vi "Preference_Panel.vi"(0 "Mode":T1) -> ()   [LabVIEW 2011]
uses:
  Anemometry Sub Vis/Controls/Server_Comms.ctl
  Anemometry Sub Vis/Controls/Preference_Mode.ctl
  Anemometry Sub Vis/File/Setup_Filetype.ctl
  Anemometry Sub Vis/Controls/Overhead.ctl
  <vilib>/Instr/_visa.llb/VISA Find Search Mode.ctl
  ADAM Client/Sub VIs/ADAM Controls/Calib_type_ADAM.ctl
  ADAM Client/Sub VIs/ADAM Controls/Module_type_ADAM.ctl
  ADAM Client/Sub VIs/ADAM Controls/Ch_description_ADAM.ctl
  ADAM Client/Sub VIs/ADAM Controls/Function_ADAM.ctl
  ADAM Client/Sub VIs/ADAM Controls/Channel_State.ctl
  ADAM Client/Sub VIs/ADAM Controls/Address.ctl
  Anemometry Sub Vis/Globals/Constants_global.vi
  Anemometry Sub Vis/Globals/Preference_global.vi
  Anemometry Sub Vis/Globals/Trav_pos_global.vi
  Anemometry Sub Vis/Globals/Qnet_Globals.vi
  Anemometry Sub Vis/Acquisition/PWA/PWAtasksGLOBAL.vi
  Anemometry Sub Vis/Globals/Dynamic_call_global.ph.vi
panel:
  in  "Post Processing Machine":bool
  in  "Analogue Device Serial No.":string="1188AB4"
  in  "PWA Device Serial No.":string="1187C98"
  in  "ADAM Setup File":u16(ring) items=["Scani_Valve.xls", "Current_Setup.xls"]
  in  "Default Source Establishment Time (s)":dbl=20.0
  out "This Machine's IP Number":string
  in  "Rig Setup":u16(ring) items=["3_x_2_tunnel", "A_Tunnel", "Adam_Sayer_Desk", "ADAM_Server", "Aero_Tunnel", "Alex_Desktop", "B_Tunnel", "Calibration_Tunnel", "Contact_Conductance", "D_Tunnel", "EnFlo_Tunnel", "Frauke_Desktop", "Fruit_Rig", "iMac_G5_2", "iMacDuo1", "Matteo's_desktop", "Matteo_PC", "Nick_PC-2", "Paul_Desk-Paul_Desk_Machine", "Paul_Hayden-Desk", "Paul_N_Desk_Machine_2", "phtest", "Post_Processing_Machine", "PowerBook_G4_1", "PowerBook_G4_2", "Syn_jet_rig", "Tank", "tdf", "Tom_Desk", "Towing_tank", "--New Rig Setup--"]
  in  "Default Traverse Name":u16(ring) items=["A_Tunnel", "Aero_Laser", "Aero_ThroughWall", "Aero_Tunnel", "Angle_Calibrator", "B_Tunnel", "D_Tunnel", "Dummy_Traverse", "EnFlo_Stack", "EnFlo_Tunnel", "EnFlo_Turntable", "Laser_Meas_Traverse", "mohd_setup", "Paul_Desk_Test", "PIV_Traverse", "--New Traverse Setup--"]
  in  "OK":bool
  in  "% Error From First Calib":dbl=10.0 format="%.1f"
  in  "% Error From Previous Calib":dbl=0.5 format="%.1f"
  in  "Qnet Site Root":path=path "/G4_2_HD/Users/paulhayden/Qnet/qnet"
  out "Templates":path=path "/G4_2_HD/Applications (Mac OS 9)/EnFlo Software/Anemometry/Anemometry Sub Vis/Templates"
  in  "Data Folder":path
  out "EnFlo SW Preferences":path=path "/G4_2_HD/Applications (Mac OS 9)/LabVIEW 5.1/EnFlo SW Preferences"
  in  "Tunnel Speed Control":bool
  in  "SMTP server IP address":string
  in  "Abs Press (mbar)":string="Froude:NPL:Atmos_Press"
  in  "Temperature":string="EnFlo Tun:Inlet Heater:Av Temp"
  in  "Server port number":u32=3363
  in  "Server address":string
  in  "LabVIEW Administrators":string[](array[string])=["", "", "", "", "", "", "", "", "", "", "", "", "", "", "", "", "", "", "", ""]
  in  "Server Comms":T2=enum."Do Not Link To Server"
  # "Server Computer Peferences"
  # "Multi Run Preferences"
  # "Warning Levels for Autocalibration Changes"
  # "Email Peferences"
  # "Deg C"
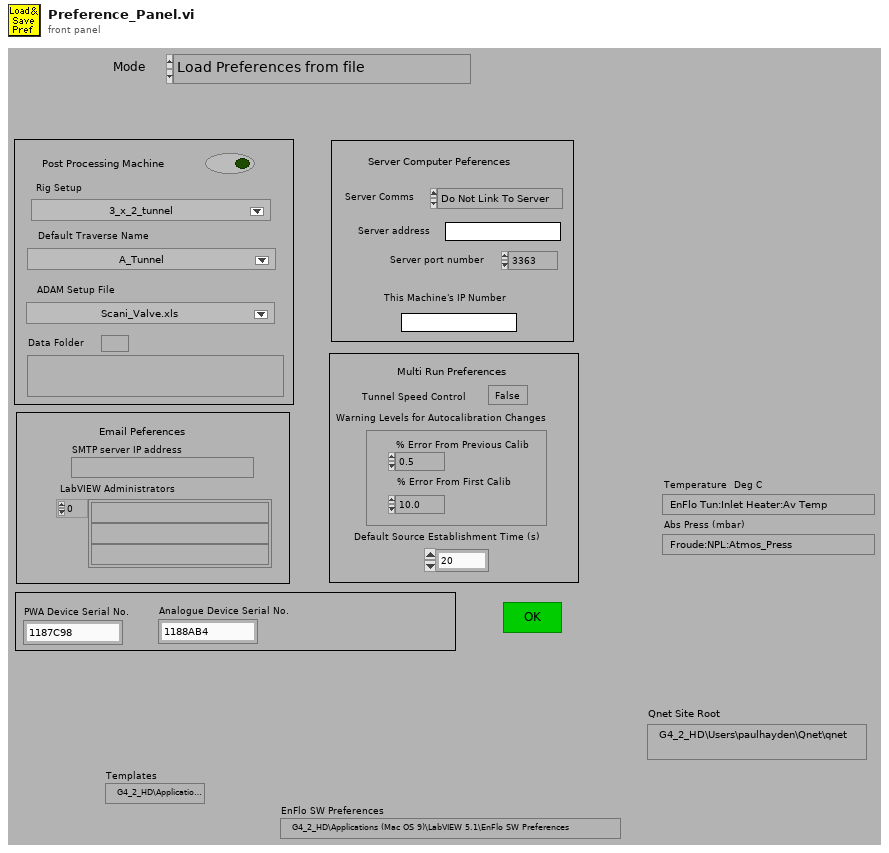
[diagram p1: front panel]
types:
  T1 = typedef "Preference_Mode.ctl" = enum16{"Load Preferences from file", "Save Preferences to file", "Load, Edit then Save"}
  T2 = typedef "Server_Comms.ctl" = enum16{"Server Link Healthy", "Do Not Link To Server"}
  T3 = enum8{"Enabled", "Disabled", "Disabled and Grayed Out"}
  T4 = enum16{"Zero or one", "One", "Zero or more", "One or more"}
  T5 = typedef "Setup_Filetype.ctl" = enum16{"Measurement Setups", "Calibration Setups", "General", "Results File Plotter Setups", "Speed Calib Tweaks"}
  T6 = typedef "Overhead.ctl" = enum16{"Update total times", "Read Current Overhead", "Re Scale totals to 3 hrs", "Initialise totals to 3hr"}
  T7 = typedef "Calib_type_ADAM.ctl" = enum16{"Raw", "Bx + A", "Cx^2 + Bx + A", "Dx^3 + Cx^2 + Bx + A", "In Band", "Hi-Tec Q", "Hi-Tec M_dot", "Text"}
  T8 = typedef "Module_type_ADAM.ctl" = enum16{"4011", "4012", "4013", "4014", "4016", "4017", "4018", "4021", "4050", "4052", "4053", "4060", "4080", "5000", "5017", "5018", "5024", "5051", "5056", "5060", "6060", "Tracker", "WEST", "GILL", "JEM", "VICI", "Vaisala", "DRUCK", "Run VI Named:", "IR2100", "PPT", "Comparator", "VIRTUAL", "Hold Value", "Read A", "Read Ch", "Coded", "Client Info", "Web Client", "X10", "Test"}
  T9 = typedef "Channel_State.ctl" = enum16{"On", "Off", "Always On", "Always Off"}
  T10 = typedef "LVDateTimeRec.ctl" = cluster{"fractional second":dbl, "second":i32, "minute":i32, "hour":i32, "day of month":i32, "month":i32, "year":i32, "day of week":i32, "day of year":i32, "DST":i32}
  T11 = typedef "VISA Find Search Mode.ctl" = u32
  T12 = typedef "Ch_description_ADAM.ctl" = cluster{"Ch Name":string, "Type":T8, "Function":T13, "Ch State":T9, "Calibration type":T7, "A":dbl, "B":dbl, "C":dbl, "D":dbl, "Comments":string, "Address":T14, "String":string, "Duty":u16}
  T13 = typedef "Function_ADAM.ctl" = enum16{"Analogue Input", "Digital Input", "Event counter", "Event rate", "Analogue Output", "Digital Output", "Relay Output"}
  T14 = typedef "Address.ctl" = cluster{"Main":i32, "Ch.":i32, "Sub":i32, "Port Name":string}
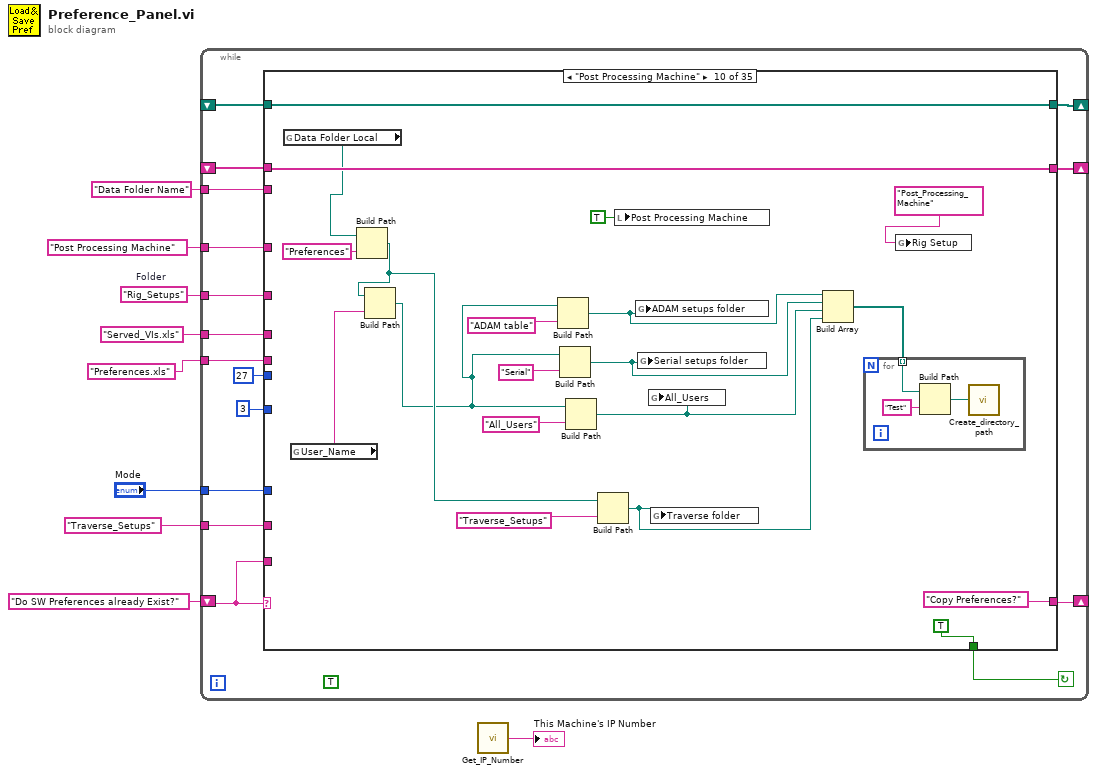
[diagram p0: block diagram]
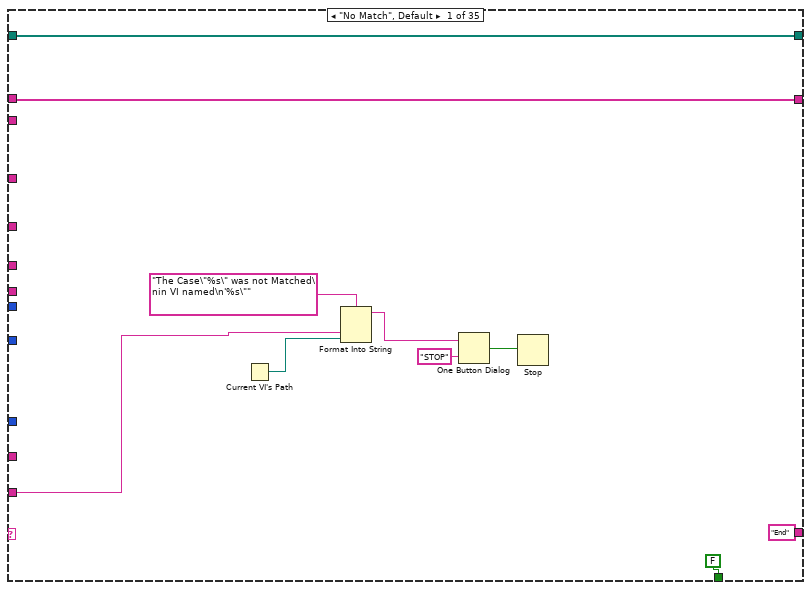
[diagram p2: hidden frame]
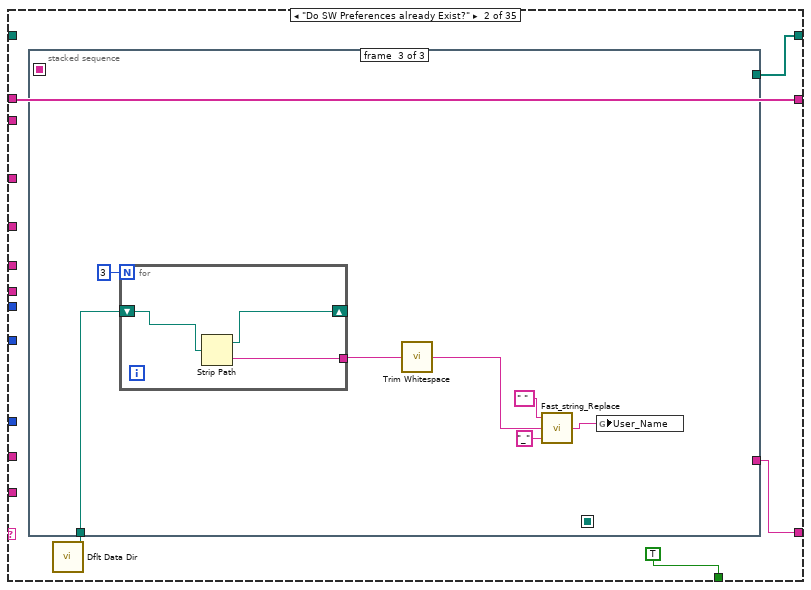
[diagram p3: hidden frame]
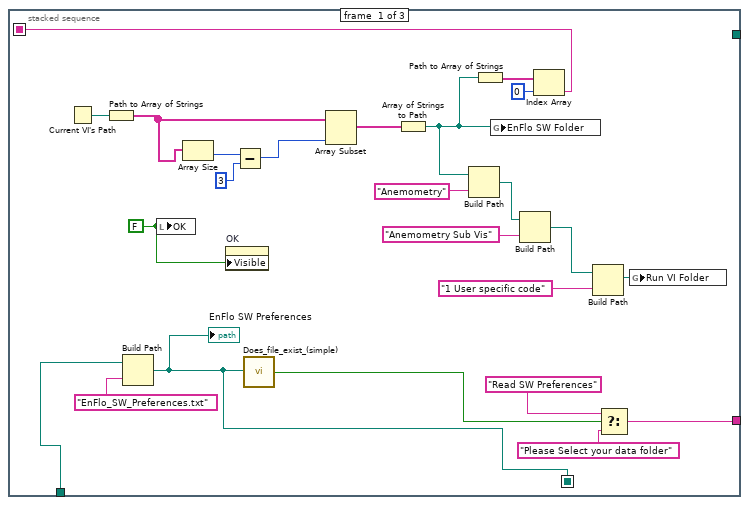
[diagram p4: hidden frame]
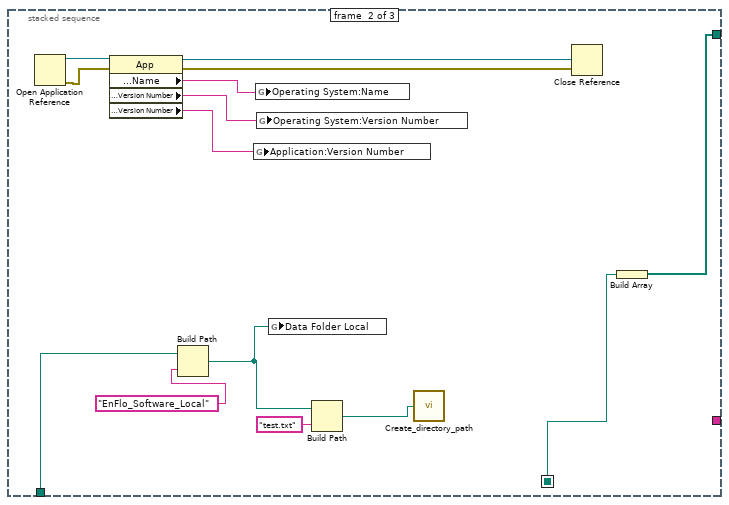
[diagram p5: hidden frame]
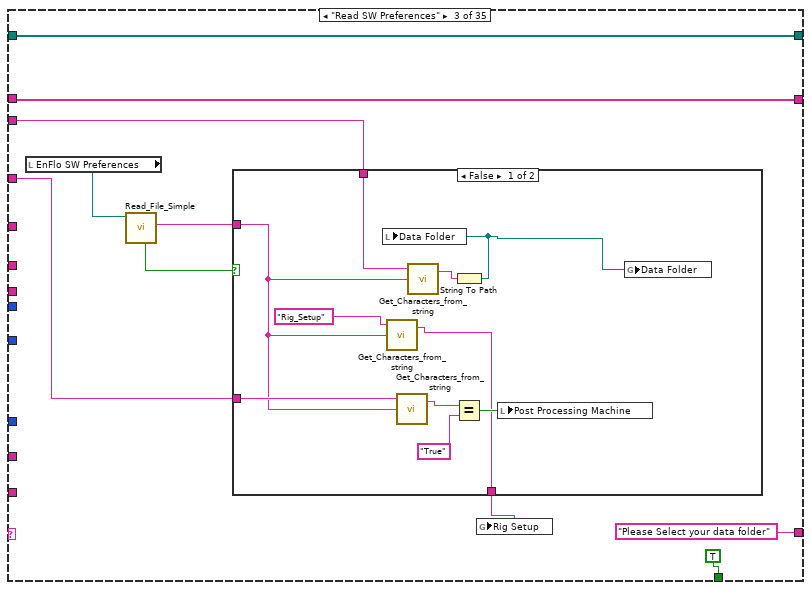
[diagram p6: hidden frame]
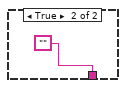
[diagram p7: hidden frame]
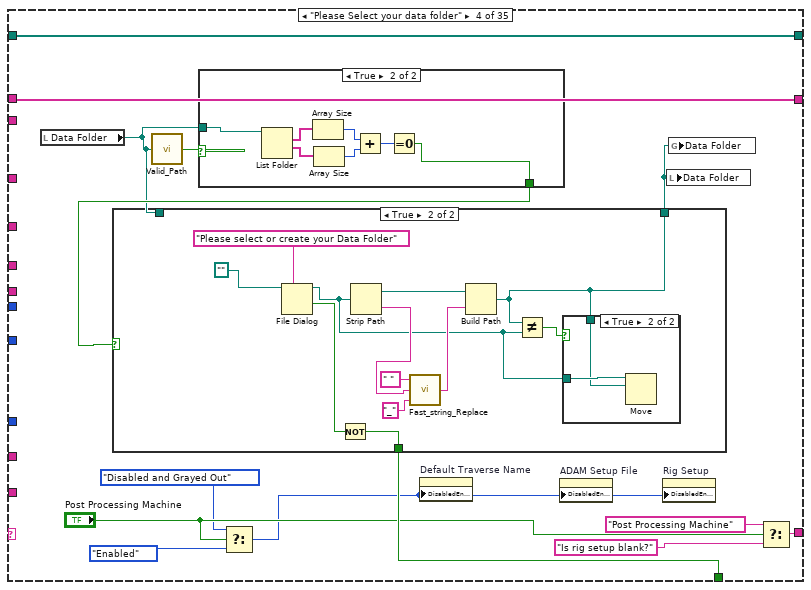
[diagram p8: hidden frame]
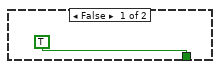
[diagram p9: hidden frame]
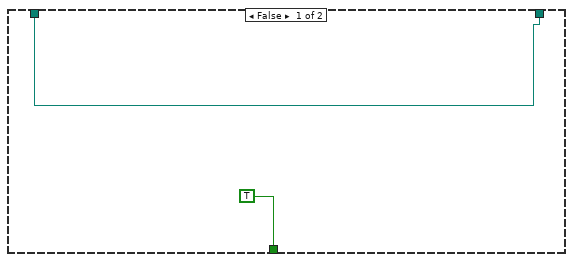
[diagram p10: hidden frame]
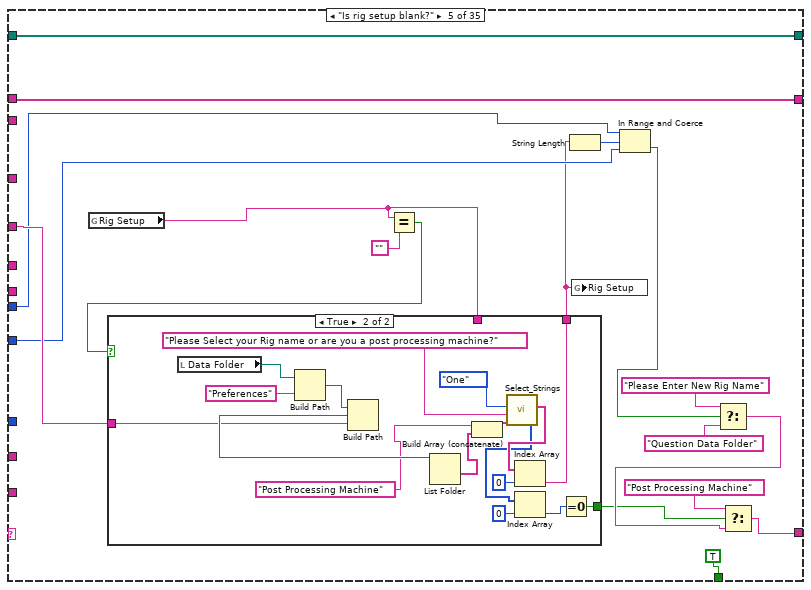
[diagram p12: hidden frame]
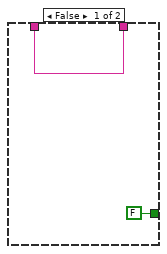
[diagram p13: hidden frame]
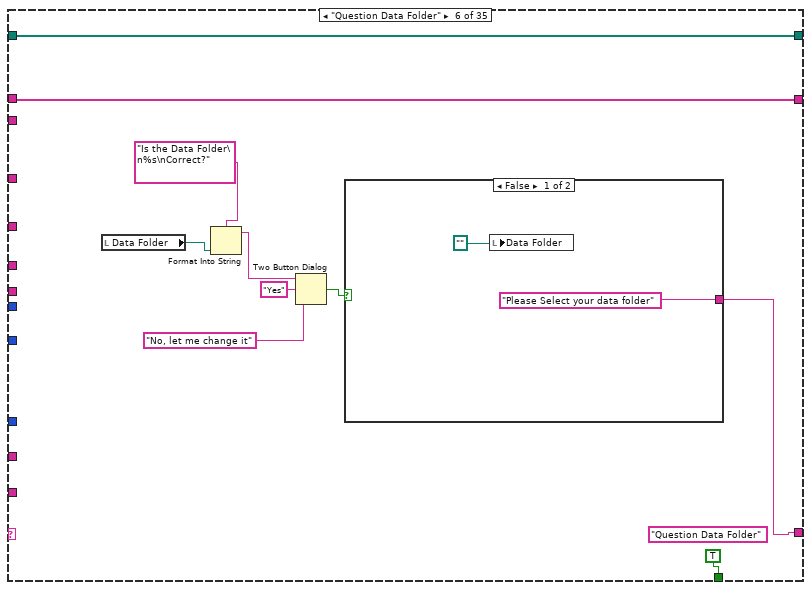
[diagram p14: hidden frame]
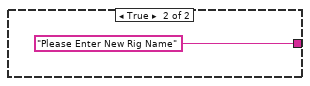
[diagram p15: hidden frame]
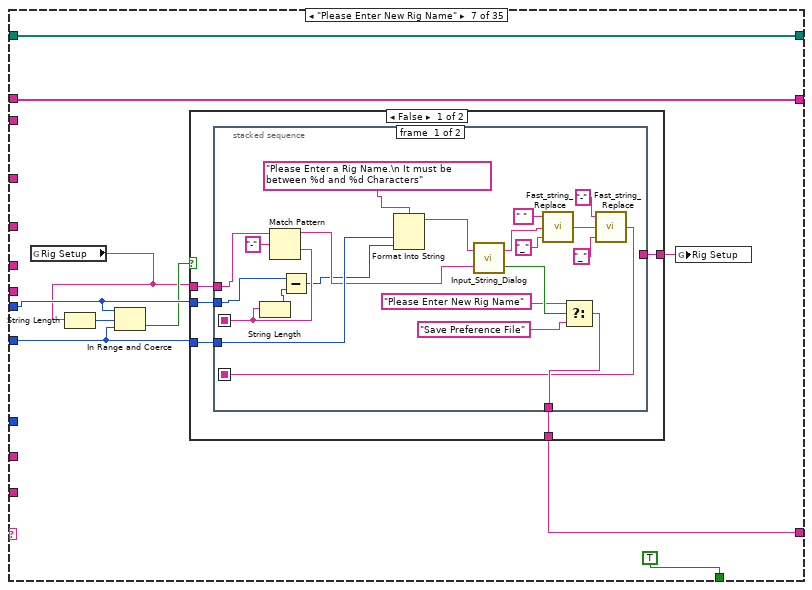
[diagram p16: hidden frame]
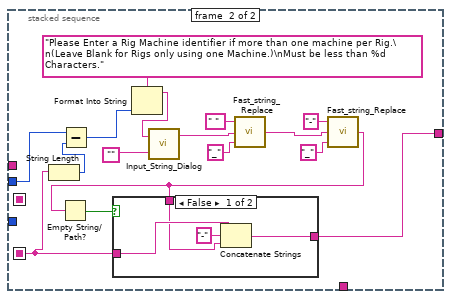
[diagram p17: hidden frame]
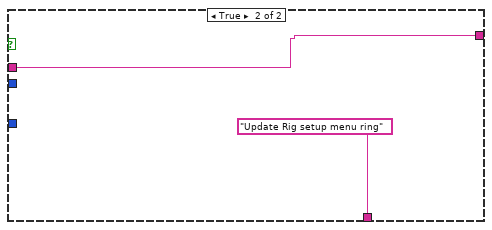
[diagram p19: hidden frame]
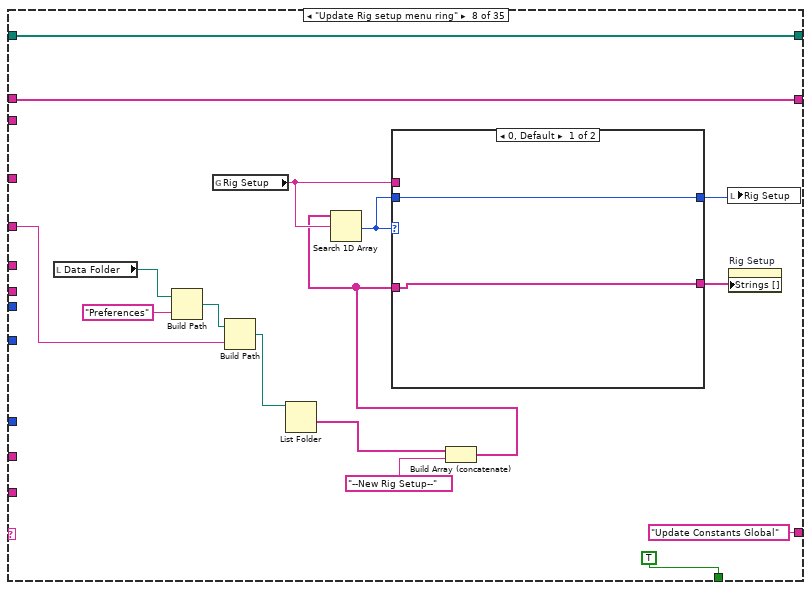
[diagram p20: hidden frame]
diagram:
  w4 = "Rig_Setups"  # Folder
  n1 = while {
    shift-left: _ -> [w22]
    shift-right: [w23] -> _
    shift-left: "Do SW Preferences already Exist?" -> [w10]
    shift-right: [w24] -> _
    tunnel: "Mode" -> [w21]
    tunnel: "Data Folder Name" ("Label for characters") -> [w20]
    tunnel: "Served_VIs.xls" ("Substring") -> [w19]
    tunnel: "Preferences.xls" ("name or relative path") -> [w18]
    tunnel: w4 -> [w15]
    tunnel: "Traverse_Setups" ("name or relative path") -> [w14]
    shift-right: [w13] -> _
    shift-left: _ -> [w12]
    tunnel: "Post Processing Machine" ("Label for characters") -> [w11]
    stop <- w25 continue-if-true
    (unwired) TRUE ("append to file? (new file:F)")
    n2 = case shown="\"Post Processing Machine\"" w10 {
      tunnel: [FALSE TRUE TRUE w117 TRUE TRUE TRUE TRUE TRUE TRUE TRUE TRUE TRUE TRUE TRUE TRUE TRUE TRUE TRUE TRUE TRUE TRUE TRUE TRUE TRUE TRUE TRUE TRUE TRUE TRUE w881 TRUE TRUE TRUE FALSE] -> w25
      tunnel: ["End" w38 "Please Select your data folder" w114 w149 w185 w204 "Update Constants Global" ("f") "Copy Preferences?" "Copy Preferences?" w332 w342 "Install Preference files" "Install Adam table files" "Install Adam setup files" "Choose ADAM Setup file" "Preference files continued" "Variable Names" w517 w537 "Please Enter new  Traverse Setup" w609 "Create Traverse setup" ("f") "Check file permission status" w706 w737 w757 w776 w793 "Save Preference File" "Save SW Preferences" w945 w958 "Initialise Globals" "End"] -> w24
      tunnel: [w27 w39 w97 w123 w164 w193 w206 w271 w297 w320 w330 w347 w405 w420 w445 w464 w486 w496 w522 w544 w597 w611 w645 w662 w707 w742 w762 w785 w798 w812 w887 w953 w959 w1011 w1071] -> w23
      tunnel: w22 -> [w27 w39 w97 w123 w164 w193 w206 w271 w297 w320 w330 w347 w405 w420 w445 w464 w486 w496 _ w544 w597 w611 w645 w662 w707 w742 w762 w785 w798 w812 w887 w953 w959 w1011 w1071]
      tunnel: w10 -> [w30 _ _ _ _ _ _ _ _ _ _ _ _ _ _ _ _ _ _ _ _ _ _ _ _ _ _ _ _ _ _ _ _ _ _]
      tunnel: w21 -> [_ _ _ _ _ _ _ _ _ _ _ _ _ _ _ _ _ _ w516 _ _ _ _ _ w705 _ _ _ _ _ w882 _ _ _ _]
      tunnel: w20 -> [_ _ w94 _ _ _ _ _ _ _ _ _ _ _ _ _ _ _ _ _ _ _ _ _ _ _ _ _ _ _ _ w944 _ _ _]
      tunnel: w19 -> [_ _ _ _ _ _ _ _ _ _ _ _ _ w415 _ _ _ _ _ _ _ _ _ _ _ _ _ _ _ _ _ _ _ w1003 _]
      tunnel: w18 -> [_ _ _ _ _ _ _ _ _ _ w326 w346 _ _ _ _ _ _ _ w534 _ _ _ _ _ _ _ _ _ _ w878 _ _ _ _]
      tunnel: 3 ("lower limit") -> [_ _ _ _ w156 _ w203 _ _ _ _ _ _ _ _ _ _ _ _ _ _ w608 _ _ _ _ _ _ _ _ _ _ _ _ _]
      tunnel: 27 ("upper limit") -> [_ _ _ _ w157 _ w202 _ _ _ _ _ _ _ _ _ _ _ _ _ _ w607 _ _ _ _ _ _ _ _ _ _ _ _ _]
      tunnel: w15 -> [_ _ _ _ w161 _ _ w259 w285 _ _ w345 _ _ _ _ _ _ _ _ _ _ _ _ _ _ _ _ _ _ _ _ _ _ _]
      tunnel: w14 -> [_ _ _ _ _ _ _ _ _ _ _ _ _ _ _ _ _ _ _ _ w595 _ w632 _ _ _ _ _ _ w811 _ _ _ _ _]
      tunnel: [w26 w36 w93 w118 w159 w192 w198 w257 w282 w309 w331 w348 w398 w411 w438 w461 w472 w488 w509 w540 w594 w603 w631 w658 path[] [] w734 w754 w779 w796 w810 w880 w941 w957 w1005 w1068] -> w13
      tunnel: w12 -> [w26 _ w93 w118 w159 w192 w198 w257 w282 w309 w331 w348 w397 w413 w438 w462 w472 w490 w509 w541 w594 w603 w631 w659 w704 w734 w754 w779 w796 w810 w880 w941 w957 w1005 w1068]
      tunnel: w11 -> [_ _ w92 _ _ _ _ _ _ _ _ _ _ _ _ _ _ _ _ _ _ _ _ _ _ _ _ _ _ _ _ w935 _ _ _]
      frame "No Match", Default {
        n3 = Current VI's Path() -> (path=w35:path)
        n4 = Format Into String(format string="The Case\"%s\" was not Matched\nin VI named\n'%s\"" ("Format String"), w30, w35) -> (resulting string=w32:string)  [unwired: 2 in, 1 out]
        n5 = One Button Dialog(message=w32, button name ("OK")="STOP") -> (true=w34:bool)
        n6 = Stop(stop? (T)=w34) -> ()
      }
      frame "Do SW Preferences already Exist?" {
        n7 = call <vilib>:"Dflt Data Dir.vi"() -> ("App:Default Data Directory"=w37:path)
        n8 = stacked-sequence {
          seq-local: [w44 _ _] -> [_ _ _]
          seq-local: [w42 _ _] -> [_ w70 _]
          tunnel: [w48 _ _] -> w38
          tunnel: w37 -> [w43 w68 w84]
          tunnel: [_ w71 _] -> w36
          frame #0 {
            w41 = FALSE ("OK")
            n9 = Current VI's Path() -> (path=w62:path)
            n10 = Path to Array of Strings(0:w62) -> (2:w59:string[])  [unwired: 1 out]
            n11 = Build Path(base path=w43, name or relative path="EnFlo_SW_Preferences.txt") -> (appended path=w42:path)
            "EnFlo SW Preferences" <- w42
            n12 = local write "OK"(w41) -> ()
            n13 = Array Size(array=w59) -> (size(s)=w61:i32)
            n14 = property on="OK" class="Bool (strict)"("Visible"=w41) -> ()  [unwired: 2 in, 2 out]
            n15 = Subtract(x=w61, y=3) -> (x-y=w57:i32)
            n16 = call "Does_file_exist_(simple).vi"("Pathname"=w42) -> ("exists?"=w63:bool)
            n17 = Array Subset(array=w59, length=w57) -> (w58:string[])  [unwired: 1 in]
            n18 = Array of Strings to Path(0:w58) -> (2:w45:path)  [unwired: 1 out]
            n19 = Build Path(base path=w45, name or relative path="Anemometry") -> (appended path=w54:path)
            n20 = Path to Array of Strings(0:w45) -> (2:w46:string[])  [unwired: 1 out]
            n21 = global write "Constants_global.vi" "EnFlo SW Folder"(w45) -> ()
            n22 = Build Path(base path=w54, name or relative path="Anemometry Sub Vis") -> (appended path=w52:path)
            n23 = Index Array(array=w46, index=0) -> (element=w44:string)
            n24 = Build Path(base path=w52, name or relative path="1 User specific code") -> (appended path=w51:path)
            n25 = Select(t="Read SW Preferences", s=w63, f="Please Select your data folder") -> (s? t:f=w48:string)
            n26 = global write "Constants_global.vi" "Run VI Folder"(w51) -> ()
          }
          frame #1 {
            n27 = Open Application Reference() -> (0:w75:errorcluster, 3:w78:refnum<vi>)  [unwired: 1 in, 3 out]
            n28 = property class="App"(reference=w78, error in=w75) -> (reference out=w77:refnum<vi>, error out=w76:errorcluster, "Operating System:Name"=w72:string, "Operating System:Version Number"=w74:string, "Application:Version Number"=w73:string)
            n29 = Build Path(base path=w68, name or relative path="EnFlo_Software_Local" ("element")) -> (appended path=w67:path)
            n30 = global write "Preference_global.vi" "Application:Version Number"(w73) -> ()
            n31 = global write "Preference_global.vi" "Operating System:Name"(w72) -> ()
            n32 = global write "Preference_global.vi" "Operating System:Version Number"(w74) -> ()
            n33 = global write "Constants_global.vi" "Data Folder Local"(w67) -> ()
            n34 = Build Path(base path=w67, name or relative path="test.txt") -> (appended path=w65:path)
            n35 = call "Create_directory_path.vi"("Path name"=w65) -> ()  [unwired: 1 out]
            n36 = Close Reference(reference=w77, error in (no error)=w76) -> ()  [unwired: 1 out]
            n37 = Build Array(w70) -> (w71:path[])
          }
          frame #2 {
            n38 = for {
              N: 3 -> [_]
              shift-right: [w88] -> _
              shift-left: w84 -> [w87]
              tunnel: [w86] -> w80
              n39 = Strip Path(path=w87) -> (stripped path=w88:path, name=w86:string)
            }
            n40 = call <vilib>:"Trim Whitespace.vi"("string"=w80) -> ("trimmed string"=w79:string)  [unwired: 1 in]
            n41 = call "Fast_string_Replace.vi"("Replace match with:"="_", "Input String"=w79, "regular expression"=" ") -> ("Output String"=w81:string)  [unwired: 1 in, 1 out]
            n42 = global write "Preference_global.vi" "User_Name"(w81) -> ()
          }
        }
      }
      frame "Read SW Preferences" {
        n43 = local read "EnFlo SW Preferences"() -> (w96:path)
        n44 = call "Read_File_Simple.vi"("Filename"=w96) -> ("Error?"=w90:bool, "string"=w91:string)  [unwired: 2 in, 6 out]
        n45 = case shown="False" w90 {
          tunnel: w94 -> [w107 _]
          tunnel: w92 -> [w104 _]
          tunnel: w91 -> [w103 _]
          tunnel: [w99 ""] -> w89
          frame False {
            n46 = call "Get_Characters_from_string.vi"("Input string"=w103, "Variable name"="Rig_Setup" ("Label for characters")) -> ("Value"=w99:string)  [unwired: 1 in, 1 out]
            n47 = call "Get_Characters_from_string.vi"("Input string"=w103, "Variable name"=w104) -> ("Value"=w102:string)  [unwired: 1 in, 1 out]
            n48 = call "Get_Characters_from_string.vi"("Input string"=w103, "Variable name"=w107) -> ("Value"=w108:string)  [unwired: 1 in, 1 out]
            n49 = String To Path(string=w108) -> (path=w106:path)
            n50 = local write "Data Folder"(w106) -> ()
            n51 = Equal?(x=w102, y="True") -> (x = y?=w100:bool)
            n52 = local write "Post Processing Machine"(w100) -> ()
            n53 = global write "Constants_global.vi" "Data Folder"(w106) -> ()
          }
          frame True {
          }
        }
        n54 = global write "Preference_global.vi" "Rig Setup"(w89) -> ()
      }
      frame "Please Select your data folder" {
        n55 = local read "Data Folder"() -> (w119:path)
        n56 = call "Valid_Path.vi"("Filename"=w119) -> ("Valid Path?"=w121:bool)
        n57 = case shown="True" w121 {
          tunnel: [TRUE ("status") w125] -> w120
          tunnel: w119 -> [_ w131]
          frame False {
          }
          frame True {
            n58 = List Folder(path=w131) -> (filenames=w129:string[], folder names=w130:string[])  [unwired: 1 in, 4 out]
            n59 = Array Size(array=w129) -> (size(s)=w127:i32)
            n60 = Array Size(array=w130) -> (size(s)=w128:i32)
            n61 = Add(x=w127, y=w128) -> (x+y=w126:i32)
            n62 = Equal To 0?(x=w126) -> (x = 0?=w125:bool)
          }
        }
        n63 = case shown="True" w120 {
          tunnel: [w133 w136] -> w122
          tunnel: w119 -> [w133 _]
          tunnel: [TRUE w134] -> w117
          frame False {
          }
          frame True {
            n64 = File Dialog(7:"Please select or create your Data Folder" ("prompt"), 11:path "") -> (1:w135:bool, 3:w137:path)  [unwired: 1 in, 6 out]
            n65 = Not(x=w135) -> (.not. x?=w134:bool)
            n66 = Strip Path(path=w137) -> (stripped path=w141:path, name=w140:string)
            n67 = call "Fast_string_Replace.vi"("Replace match with:"="_", "Input String"=w140, "regular expression"=" ") -> ("Output String"=w139:string)  [unwired: 2 out]
            n68 = Build Path(base path=w141, name or relative path=w139) -> (appended path=w136:path)
            n69 = Not Equal?(x=w136, y=w137) -> (x != y?=w138:bool)
            n70 = case shown="True" w138 {
              tunnel: w137 -> [_ w147]
              tunnel: w136 -> [_ w146]
              frame False {
              }
              frame True {
                n71 = Move(source path=w147, 10:w146) -> ()  [unwired: 1 in, 5 out]
              }
            }
          }
        }
        n72 = Select(t=T3."Disabled and Grayed Out" ("Disabled"), s="Post Processing Machine", f=T3."Enabled" ("Disabled")) -> (s? t:f=w110:T3)
        n73 = property on="Default Traverse Name" class="Ring (strict)"("DisabledEnum"=w110) -> ()  [unwired: 2 in, 2 out]
        n74 = property on="ADAM Setup File" class="Ring (strict)"("DisabledEnum"=w110) -> ()  [unwired: 2 in, 2 out]
        n75 = property on="Rig Setup" class="Ring (strict)"("DisabledEnum"=w110) -> ()  [unwired: 2 in, 2 out]
        n76 = local write "Data Folder"(w122) -> ()
        n77 = global write "Constants_global.vi" "Data Folder"(w122) -> ()
        n78 = Select(t="Post Processing Machine", s="Post Processing Machine", f="Is rig setup blank?") -> (s? t:f=w114:string)
      }
      frame "Is rig setup blank?" {
        n79 = global read "Preference_global.vi" "Rig Setup"() -> (w160:string)
        n80 = Equal?(x=w160, y="") -> (x = y?=w162:bool)
        n81 = case shown="True" w162 {
          tunnel: w161 -> [_ w180]
          tunnel: [w167 w178] -> w155
          tunnel: w160 -> [w167 _]
          tunnel: [FALSE w168] -> w148
          frame False {
          }
          frame True {
            n82 = local read "Data Folder"() -> (w183:path)
            n83 = Build Path(base path=w183, name or relative path="Preferences") -> (appended path=w182:path)
            n84 = Build Path(base path=w182, name or relative path=w180) -> (appended path=w181:path)
            n85 = List Folder(path=w181) -> (folder names=w175:string[])  [unwired: 1 in, 5 out]
            n86 = Build Array (concatenate)("Post Processing Machine", w175) -> (w173:string[])
            n87 = call "Select_Strings.vi"("Available Ch names"=w173, "Message"="Please Select your Rig name or are you a post processing machine?", "Selector mode"=T4."One") -> ("Ch Indicies Choosen"=w170:i32[], "Selected Channel Names"=w172:string[])  [unwired: 3 in, 1 out]
            n88 = Index Array(array=w172, index=0) -> (element=w178:string)
            n89 = Index Array(array=w170, index=0) -> (element=w169:i32)
            n90 = Equal To 0?(x=w169) -> (x = 0?=w168:bool)
          }
        }
        n91 = String Length(string=w155) -> (length=w158:i32)
        n92 = global write "Preference_global.vi" "Rig Setup"(w155) -> ()
        n93 = In Range and Coerce(upper limit=w157, x=w158, lower limit=w156) -> (In Range?=w154:bool)  [unwired: 1 out]
        n94 = Select(t="Please Enter New Rig Name", s=w154, f="Question Data Folder") -> (s? t:f=w150:string)
        n95 = Select(t="Post Processing Machine", s=w148, f=w150) -> (s? t:f=w149:string)
      }
      frame "Question Data Folder" {
        (unwired) "Question Data Folder"
        n96 = local read "Data Folder"() -> (w191:path)
        n97 = Format Into String(format string="Is the Data Folder\n%s\nCorrect?" ("message"), w191) -> (resulting string=w189:string)  [unwired: 2 in, 1 out]
        n98 = Two Button Dialog(message=w189, 1:"No, let me change it" ("F button name (\"Cancel\")"), 2:"Yes" ("T button name (\"OK\")")) -> (T button?=w186:bool)
        n99 = case shown="False" w186 {
          tunnel: ["Please Select your data folder" "Please Enter New Rig Name"] -> w185
          frame False {
            n100 = local write "Data Folder"(path "") -> ()
          }
          frame True {
          }
        }
      }
      frame "Please Enter New Rig Name" {
        n101 = global read "Preference_global.vi" "Rig Setup"() -> (w200:string)
        n102 = String Length(string=w200) -> (length=w205:i32)
        n103 = In Range and Coerce(upper limit=w202, x=w205, lower limit=w203) -> (In Range?=w201:bool)  [unwired: 1 out]
        n104 = case shown="False" w201 {
          tunnel: w200 -> [w212 w255]
          tunnel: [w208 "Update Rig setup menu ring"] -> w204
          tunnel: [w209 w255] -> w199
          tunnel: w203 -> [w211 _]
          tunnel: w202 -> [w210 _]
          frame False {
            n105 = stacked-sequence {
              seq-local: [w213 _] -> [_ w238]
              seq-local: [w220 _] -> [_ _]
              tunnel: w212 -> [w222 _]
              tunnel: w211 -> [w233 _]
              tunnel: w210 -> [w219 w236]
              tunnel: [_ w241] -> w209
              tunnel: [w225 _] -> w208
              frame #0 {
                n106 = Match Pattern(string=w222, regular expression="-") -> (before substring=w221:string, after substring=w220:string)  [unwired: 3 out]
                n107 = String Length(string=w220) -> (length=w218:i32)
                n108 = Subtract(x=w219, y=w218) -> (x-y=w217:i32)
                n109 = Format Into String(format string="Please Enter a Rig Name.\n It must be between %d and %d Characters" ("Message to user"), w233, w217) -> (resulting string=w232:string)  [unwired: 2 in, 1 out]
                n110 = call "Input_String_Dialog.vi"("Value"=w221, "Message to user"=w232) -> ("Ok Out"=w228:bool, "Output string"=w229:string)
                n111 = call "Fast_string_Replace.vi"("Replace match with:"="_", "Input String"=w229, "regular expression"=" ") -> ("Output String"=w214:string)  [unwired: 2 out]
                n112 = Select(t="Please Enter New Rig Name", s=w228, f="Save Preference File") -> (s? t:f=w225:string)
                n113 = call "Fast_string_Replace.vi"("Replace match with:"="_", "Input String"=w214, "regular expression"="-") -> ("Output String"=w213:string)  [unwired: 2 out]
              }
              frame #1 {
                n114 = String Length(string=w238) -> (length=w237:i32)
                n115 = Subtract(x=w236, y=w237) -> (x-y=w235:i32)
                n116 = Format Into String(format string="Please Enter a Rig Machine identifier if more than one machine per Rig.\n(Leave Blank for Rigs only using one Machine.)\nMust be less than %d Characters." ("Message to user"), w235) -> (resulting string=w234:string)  [unwired: 2 in, 1 out]
                n117 = call "Input_String_Dialog.vi"("Value"="", "Message to user"=w234) -> ("Output string"=w247:string)  [unwired: 1 out]
                n118 = call "Fast_string_Replace.vi"("Replace match with:"="_", "Input String"=w247, "regular expression"=" ") -> ("Output String"=w243:string)  [unwired: 2 out]
                n119 = call "Fast_string_Replace.vi"("Replace match with:"="_", "Input String"=w243, "regular expression"="-") -> ("Output String"=w240:string)  [unwired: 2 out]
                n120 = Empty String/Path?(string/path=w240) -> (empty?=w242:bool)
                n121 = case shown="False" w242 {
                  tunnel: [w250 w254] -> w241
                  tunnel: w238 -> [w253 w254]
                  tunnel: w240 -> [w251 _]
                  frame False {
                    n122 = Concatenate Strings(w253, "-" ("string"), w251) -> (w250:string)
                  }
                  frame True {
                  }
                }
              }
            }
          }
          frame True {
          }
        }
        n123 = global write "Preference_global.vi" "Rig Setup"(w199) -> ()
      }
      frame "Update Rig setup menu ring" {
        n124 = local read "Data Folder"() -> (w262:path)
        n125 = Build Path(base path=w262, name or relative path="Preferences") -> (appended path=w261:path)
        n126 = global read "Preference_global.vi" "Rig Setup"() -> (w268:string)
        n127 = Build Path(base path=w261, name or relative path=w259) -> (appended path=w260:path)
        n128 = List Folder(path=w260) -> (folder names=w258:string[])  [unwired: 1 in, 5 out]
        n129 = Build Array (concatenate)(w258, "--New Rig Setup--") -> (w264:string[])
        n130 = Search 1D Array(1D array=w264, element=w268) -> (index of element=w267:i32)  [unwired: 1 out]
        n131 = case shown="0, Default" w267 {
          tunnel: [w274 0] -> w270
          tunnel: w264 -> [w273 w277]
          tunnel: w268 -> [_ w276]
          tunnel: w267 -> [w274 _]
          tunnel: [w273 w275] -> w266
          frame 0, Default {
          }
          frame -1 {
            n132 = Build Array (concatenate)(w276, w277) -> (w275:string[])
          }
        }
        n133 = local write "Rig Setup"(w270) -> ()
        n134 = property on="Rig Setup" class="Ring (strict)"("Strings []"=w266) -> ()  [unwired: 2 in, 2 out]
      }
      frame "Update Constants Global" {
        n135 = global read "Constants_global.vi" "Data Folder"() -> (w283:path)
        n136 = global read "Preference_global.vi" "Rig Setup"() -> (w284:string)
        n137 = Build Path(base path=w283, name or relative path="Preferences") -> (appended path=w286:path)
        n138 = Build Path(base path=w286, name or relative path=w285) -> (appended path=w287:path)
        n139 = Build Path(base path=w287, name or relative path=w284) -> (appended path=w279:path)
        n140 = Build Path(base path=w279, name or relative path="ADAM table") -> (appended path=w292:path)
        n141 = Build Path(base path=w279, name or relative path="Serial") -> (appended path=w291:path)
        n142 = Build Path(base path=w279, name or relative path="All_Users") -> (appended path=w280:path)
        n143 = Build Path(base path=w286, name or relative path="Traverse_Setups") -> (appended path=w290:path)
        n144 = global write "Constants_global.vi" "ADAM setups folder"(w292) -> ()
        n145 = global write "Constants_global.vi" "Serial setups folder"(w291) -> ()
        n146 = global write "Constants_global.vi" "All_Users"(w280) -> ()
        n147 = global write "Constants_global.vi" "Traverse folder"(w290) -> ()
        n148 = Build Array(w292, w291, w280, w290) -> (w289:path[])
        n149 = for {
          tunnel: w289 -> [w301] mode=indexing
          n150 = Build Path(base path=w301, name or relative path="Test") -> (appended path=w299:path)
          n151 = call "Create_directory_path.vi"("Path name"=w299) -> ()  [unwired: 1 out]
        }
      }
      frame "Post Processing Machine" {
        n152 = global read "Constants_global.vi" "Data Folder Local"() -> (w308:path)
        n153 = global read "Preference_global.vi" "User_Name"() -> (w303:string)
        n154 = Build Path(base path=w308, name or relative path="Preferences") -> (appended path=w310:path)
        n155 = Build Path(base path=w310, name or relative path=w303) -> (appended path=w304:path)
        n156 = Build Path(base path=w304, name or relative path="ADAM table") -> (appended path=w315:path)
        n157 = Build Path(base path=w304, name or relative path="Serial") -> (appended path=w314:path)
        n158 = Build Path(base path=w304, name or relative path="All_Users") -> (appended path=w305:path)
        n159 = Build Path(base path=w310, name or relative path="Traverse_Setups") -> (appended path=w313:path)
        n160 = local write "Post Processing Machine"(TRUE ("Post Processing Machine")) -> ()
        n161 = global write "Constants_global.vi" "ADAM setups folder"(w315) -> ()
        n162 = global write "Constants_global.vi" "Serial setups folder"(w314) -> ()
        n163 = global write "Constants_global.vi" "All_Users"(w305) -> ()
        n164 = global write "Constants_global.vi" "Traverse folder"(w313) -> ()
        n165 = Build Array(w315, w314, w305, w313) -> (w312:path[])
        n166 = for {
          tunnel: w312 -> [w324] mode=indexing
          n167 = Build Path(base path=w324, name or relative path="Test") -> (appended path=w322:path)
          n168 = call "Create_directory_path.vi"("Path name"=w322) -> ()  [unwired: 1 out]
        }
        n169 = global write "Preference_global.vi" "Rig Setup"("Post_Processing_Machine" ("Rig Setup")) -> ()
      }
      frame "Copy Preferences?" {
        n170 = call "Setup_Filepath.vi"("Setup File Type"=Setup_Filetype."General", "Filename in"=w326) -> ("Filename Out"=w325:path)  [unwired: 1 out]
        n171 = call <vilib>:"Check if File or Folder Exists.vi"("path"=w325) -> ("file or folder exists?"=w329:bool)  [unwired: 1 in, 9 out]
        n172 = case shown="False" w329 {
          tunnel: [w336 TRUE ("Error?")] -> w328
          frame False {
            n173 = global read "Constants_global.vi" "All_Users"() -> (w338:path)
            n174 = Build Path(base path=w338, name or relative path="Current_Username") -> (appended path=w339:path)
            n175 = call "Read_File_Simple.vi"("Filename"=w339) -> ("Error?"=w336:bool)  [unwired: 4 in, 5 out]
          }
          frame True {
          }
        }
        n176 = Select(t="Install Generic Meas Setup file", s=w328, f="Copy from last user") -> (s? t:f=w332:string)
      }
      frame "Copy from last user" {
        n177 = stacked-sequence {
          seq-local: [w359 _ _ _] -> [_ w369 w378 w390]
          seq-local: [_ w364 _ _] -> [_ _ _ w384]
          seq-local: [_ _ w373 _] -> [_ _ _ w383]
          tunnel: w346 -> [_ w367 _ _]
          tunnel: w345 -> [_ _ _ _]
          tunnel: [_ _ _ w382] -> w344
          frame #0 {
            n178 = global read "Constants_global.vi" "All_Users"() -> (w363:path)
            n179 = Seconds To Date/Time() -> (date time rec=w354:T10)  [unwired: 2 out]
            n180 = Unbundle By Name(w354) -> ("year"=w355:i32)
            n181 = global read "Preference_global.vi" "Rig Setup"() -> (w352:string)
            n182 = Build Path(base path=w363, name or relative path="Current_Username") -> (appended path=w361:path)
            n183 = Number To Decimal String(number=w355) -> (decimal integer string=w353:string)  [unwired: 1 out]
            n184 = global read "Constants_global.vi" "Data Folder"() -> (w358:path)
            n185 = call "Read_File_Simple.vi"("Filename"=w361) -> ("string"=w351:string)  [unwired: 4 in, 5 out]
            n186 = Build Path(base path=w358, name or relative path=w353) -> (appended path=w357:path)
            n187 = Build Path(base path=w357, name or relative path=w352) -> (appended path=w356:path)
            n188 = Build Path(base path=w356, name or relative path=w351) -> (appended path=w360:path)
            n189 = Build Path(base path=w360, name or relative path="Preferences") -> (appended path=w359:path)
          }
          frame #1 {
            n190 = call "Setup_Filepath.vi"("Setup File Type"=Setup_Filetype."General", "Filename in"=w367) -> ("Filename Out"=w366:path)  [unwired: 1 out]
            n191 = Build Path(base path=w369, name or relative path="General") -> (appended path=w371:path)
            n192 = Build Path(base path=w371, name or relative path=w367) -> (appended path=w370:path)
            n193 = Copy(10:w366, 11:w370) -> (0:w365:errorcluster)  [unwired: 3 in, 2 out]
            n194 = Unbundle By Name(w365) -> ("status"=w364:bool)
          }
          frame #2 {
            w376 = "Current_Setup.xls"
            n195 = Build Path(base path=w378, name or relative path="Meas Setups") -> (appended path=w380:path)
            n196 = Build Path(base path=w380, name or relative path=w376) -> (appended path=w379:path)
            n197 = call "Setup_Filepath.vi"("Setup File Type"=Setup_Filetype."Measurement Setups", "Filename in"=w376) -> ("Filename Out"=w375:path)  [unwired: 1 out]
            n198 = Copy(10:w375, 11:w379) -> (0:w374:errorcluster)  [unwired: 3 in, 2 out]
            n199 = Unbundle By Name(w374) -> ("status"=w373:bool)
          }
          frame #3 {
            w388 = "Current_Setup.xls"
            n200 = Build Path(base path=w390, name or relative path="Calib Setups") -> (appended path=w392:path)
            n201 = Build Path(base path=w392, name or relative path=w388) -> (appended path=w391:path)
            n202 = call "Setup_Filepath.vi"("Setup File Type"=Setup_Filetype."Calibration Setups", "Filename in"=w388) -> ("Filename Out"=w387:path)  [unwired: 1 out]
            n203 = Copy(10:w387, 11:w391) -> (0:w386:errorcluster)  [unwired: 3 in, 2 out]
            n204 = Unbundle By Name(w386) -> ("status"=w385:bool)
            n205 = Compound Arithmetic op=OR(w385, w384, w383) -> (w382:bool)
          }
        }
        n206 = Select(t="Install Generic Meas Setup file", s=w344, f="Read SW Preferences") -> (s? t:f=w342:string)
      }
      frame "Install Generic Meas Setup file" {
        n207 = global read "Constants_global.vi" "Run VI Folder"() -> (w404:path)
        n208 = Strip Path(path=w404) -> (stripped path=w402:path)  [unwired: 1 out]
        n209 = call "Setup_Filepath.vi"("Setup File Type"=Setup_Filetype."Measurement Setups", "Filename in"="Current_Setup.xls" ("name or relative path")) -> ("Filename Out"=w394:path)  [unwired: 1 out]
        n210 = Build Path(base path=w402, name or relative path="Templates") -> (appended path=w400:path)
        "Templates" <- w400
        n211 = call "Does_file_exist_(simple).vi"("Pathname"=w394) -> ("exists?"=w401:bool)
        n212 = case shown="False" w401 {
          tunnel: w394 -> [w410 _]
          tunnel: w400 -> [w408 _]
          frame False {
            n213 = Build Path(base path=w408, name or relative path="Measurement Setup.xls") -> (appended path=w407:path)
            n214 = Copy(10:w410, 11:w407) -> ()  [unwired: 1 in, 5 out]
          }
          frame True {
          }
        }
        n215 = Build Array (concatenate)(w397, w394) -> (w398:path[])
      }
      frame "Install Preference files" {
        n216 = Build Array("Preferences.xls" ("Substring"), w415, "Month_Names.xls" ("name or relative path"), "LDA_Configuration.xls") -> (w419:string[])
        n217 = for {
          tunnel: w419 -> [w423] mode=indexing
          tunnel: [w422] -> w412 mode=indexing
          n218 = call "Setup_Filepath.vi"("Setup File Type"=Setup_Filetype."General", "Filename in"=w423) -> ("Filename Out"=w422:path)  [unwired: 1 out]
          n219 = call "Does_file_exist_(simple).vi"("Pathname"=w422) -> ("exists?"=w425:bool)
          n220 = case shown="False" w425 {
            tunnel: w422 -> [w429 _]
            tunnel: w423 -> [w426 _]
            frame False {
              n221 = local read "Templates"() -> (w427:path)
              n222 = Build Path(base path=w427, name or relative path=w426) -> (appended path=w428:path)
              n223 = Copy(10:w429, 11:w428) -> ()  [unwired: 1 in, 5 out]
            }
            frame True {
            }
          }
        }
        n224 = Build Array (concatenate)(w413, w412) -> (w411:path[])
      }
      frame "Install Adam table files" {
        w434 = "Current_Setup.xls"
        n225 = global read "Constants_global.vi" "ADAM setups folder"() -> (w436:path)
        n226 = Build Path(base path=w436, name or relative path=w434) -> (appended path=w437:path)
        n227 = Build Path(base path=w436, name or relative path="Setup_Files") -> (appended path=w432:path)
        n228 = Build Array("Hi_Tec_Calibs.xls" ("name or relative path"), "A_Tunnel DB setup.xls" ("Substring"), "EnFlo_Tunnel DB setup.xls", "Aero_Tunnel DB setup.xls" ("name or relative path"), "D_Tunnel DB setup.xls") -> (w444:string[])
        n229 = Build Path(base path=w432, name or relative path=w434) -> (appended path=w431:path)
        n230 = for {
          tunnel: w444 -> [w448] mode=indexing
          tunnel: w436 -> [w449]
          n231 = Build Path(base path=w449, name or relative path=w448) -> (appended path=w447:path)
          n232 = call "Does_file_exist_(simple).vi"("Pathname"=w447) -> ("exists?"=w450:bool)
          n233 = case shown="False" w450 {
            tunnel: w447 -> [w454 _]
            tunnel: w448 -> [w451 _]
            frame False {
              n234 = local read "Templates"() -> (w452:path)
              n235 = Build Path(base path=w452, name or relative path=w451) -> (appended path=w453:path)
              n236 = Copy(10:w454, 11:w453) -> ()  [unwired: 1 in, 5 out]
            }
            frame True {
            }
          }
        }
        n237 = call "Create_directory_path.vi"("Path name"=w431) -> ("Path name Out"=w430:path)
        n238 = Move(source path=w437, 10:w430) -> ()  [unwired: 1 in, 5 out]
      }
      frame "Install Adam setup files" {
        w458 = "Current_Setup.xls"
        n239 = global read "Constants_global.vi" "ADAM setups folder"() -> (w460:path)
        n240 = Build Path(base path=w460, name or relative path="Setup_Files") -> (appended path=w457:path)
        n241 = Build Path(base path=w457, name or relative path=w458) -> (appended path=w455:path)
        n242 = call "Does_file_exist_(simple).vi"("Pathname"=w455) -> ("exists?"=w456:bool)
        n243 = case shown="False" w456 {
          tunnel: w455 -> [w471 _]
          tunnel: w458 -> [w469 _]
          frame False {
            n244 = local read "Templates"() -> (w470:path)
            n245 = Build Path(base path=w470, name or relative path="ADAM_Setup_files") -> (appended path=w468:path)
            n246 = Build Path(base path=w468, name or relative path=w469) -> (appended path=w467:path)
            n247 = Copy(10:w471, 11:w467) -> ()  [unwired: 1 in, 5 out]
          }
          frame True {
          }
        }
        n248 = Build Array (concatenate)(w462, w455) -> (w461:path[])
      }
      frame "Choose ADAM Setup file" {
        w480 = "Selected_Filename.txt" ("Substring")
        n249 = global read "Constants_global.vi" "ADAM setups folder"() -> (w484:path)
        n250 = Build Path(base path=w484, name or relative path="Setup_Files") -> (appended path=w481:path)
        n251 = Build Path(base path=w481, name or relative path=w480) -> (appended path=w479:path)
        n252 = call "Read_File_Simple.vi"("Filename"=w479) -> ("string"=w477:string)  [unwired: 2 in, 7 out]
        n253 = Build Array(w480) -> (w482:string[])
        n254 = call "List_files_in_order_of_age.vi"("Files to Hide"=w482, "Folder"=w481) -> ("file names"=w478:string[])
        n255 = Search 1D Array(1D array=w478, element=w477) -> (index of element=w474:i32)  [unwired: 1 out]
        n256 = property on="ADAM Setup File" class="Ring (strict)"("Strings []"=w478) -> ()  [unwired: 2 in, 2 out]
        n257 = Less Than 0?(x=w474) -> (x < 0?=w475:bool)
        n258 = Select(t=0, s=w475, f=w474) -> (s? t:f=w473:i32)
        n259 = local write "ADAM Setup File"(w473) -> ()
      }
      frame "Preference files continued" {
        n260 = Build Array("Hot_Wire_Bridges.txt", "Hot_Wire_Probes.txt", "Pressure_Transducers.txt") -> (w491:string[])
        n261 = for {
          tunnel: w491 -> [w499] mode=indexing
          tunnel: [w498] -> w489 mode=indexing
          n262 = call "Setup_Filepath.vi"("Setup File Type"=Setup_Filetype."Calibration Setups", "Filename in"=w499) -> ("Filename Out"=w498:path)  [unwired: 1 out]
          n263 = call "Does_file_exist_(simple).vi"("Pathname"=w498) -> ("exists?"=w501:bool)
          n264 = case shown="False" w501 {
            tunnel: w498 -> [w505 _]
            tunnel: w499 -> [w502 _]
            frame False {
              n265 = local read "Templates"() -> (w503:path)
              n266 = Build Path(base path=w503, name or relative path=w502) -> (appended path=w504:path)
              n267 = Copy(10:w505, 11:w504) -> ()  [unwired: 1 in, 5 out]
            }
            frame True {
            }
          }
        }
        n268 = Build Array (concatenate)(w490, w489) -> (w488:path[])
      }
      frame "Variable Names" {
        n269 = Build Array("PWA Device Serial No.", "Analogue Device Serial No.", "Server address", "Server port number", "LabVIEW Administrators", "SMTP server IP address", "Server Comms", "Default Source Establishment Time (s)", "Temperature", "Abs Press (mbar)", "Default Traverse Name", "Tunnel Speed Control", "Current Overhead Factor", "Qnet Site Root", "Auto Calib Error fr Previous", "Auto Calib Error fr First") -> (w522:string[])
        n270 = case shown="\"Load, Edit then Save\"" w516 {
          tunnel: ["Load From Preference file" w528 "Save Preference File"] -> w517
          frame "Load Preferences from file" {
          }
          frame "Load, Edit then Save" {
            n271 = local read "OK"() -> (w531:bool)
            n272 = Select(t="Save Preference File", s=w531, f="Load From Preference file") -> (s? t:f=w528:string)
          }
          frame "Save Preferences to file" {
          }
        }
      }
      frame "Load From Preference file" {
        n273 = call "Setup_Filepath.vi"("Setup File Type"=Setup_Filetype."General", "Filename in"=w534) -> ("Filename Out"=w533:path)  [unwired: 1 out]
        n274 = call "Read_File_Simple.vi"("Filename"=w533) -> ("string"=w542:string)  [unwired: 2 in, 7 out]
        n275 = for {
          tunnel: w544 -> [w547] mode=indexing
          tunnel: w542 -> [w546]
          w549 = FALSE  # Show Dialog?
          n276 = call "Get_Characters_from_string.vi"("Show Dialog?"=w549, "Input string"=w546, "Variable name"=w547) -> ("Status"=w548:enum16{"Char in string", "Char not in string"}, "Value"=w545:string)
          n277 = case shown="\"Char in string\"" w548 {
            tunnel: w547 -> [w551 _]
            tunnel: w545 -> [w550 _]
            frame "Char in string" {
              n278 = case shown="\"Server address\"" w551 {
                tunnel: w551 -> [w553 _ _ _ _ _ _ _ _ _ _ _ _ _ _ _ _]
                tunnel: w550 -> [_ w554 w555 w558 w559 w560 w562 w564 w567 _ w571 w575 w576 w578 w580 w583 w585]
                tunnel: w550 -> [_ _ _ _ _ _ _ _ _ w568 _ _ _ _ _ _ _]
                frame "No Match", Default {
                  n279 = call "Was_string_matched.vi"("Match Error"=TRUE, "Variable name"=w553) -> ()  [unwired: 1 in]
                }
                frame "Server address" {
                  n280 = global write "Preference_global.vi" "Server address"(w554) -> ()
                  n281 = local write "Server address"(w554) -> ()
                }
                frame "Default Traverse Name" {
                  n282 = global write "Trav_pos_global.vi" "Default Traverse Setup"(w555) -> ()
                }
                frame "Server port number" {
                  n283 = Decimal String To Number(string=w558) -> (number=w557:i32)  [unwired: 3 out]
                  n284 = To Unsigned Long Integer(number=w557) -> (unsigned 32bit integer=w556:u32)
                  n285 = local write "Server port number"(w556) -> ()
                  n286 = global write "Preference_global.vi" "Server port number"(w556) -> ()
                }
                frame "Analogue Device Serial No." {
                  n287 = local write "Analogue Device Serial No."(w559) -> ()
                }
                frame "PWA Device Serial No." {
                  n288 = local write "PWA Device Serial No."(w560) -> ()
                }
                frame "Default Source Establishment Time (s)" {
                  n289 = Fract/Exp String To Number(string=w562) -> (number=w561:dbl)  [unwired: 4 out]
                  n290 = global write "Preference_global.vi" "Default Source Establishment Time (s)"(w561) -> ()
                  n291 = local write "Default Source Establishment Time (s)"(w561) -> ()
                }
                frame "Tunnel Speed Control" {
                  n292 = Equal?(x="TRUE", y=w564) -> (x = y?=w563:bool)
                  n293 = local write "Tunnel Speed Control"(w563) -> ()
                  n294 = global write "Preference_global.vi" "Tunnel Speed Control"(w563) -> ()
                }
                frame "LabVIEW Administrators" {
                  n295 = call "Get_array_values_fr_String.vi"("String Value"=w567) -> ("String array"=w566:string[])  [unwired: 1 out]
                  n296 = global write "Preference_global.vi" "LabVIEW Administrators"(w566) -> ()
                  n297 = local write "LabVIEW Administrators"(w566) -> ()
                }
                frame "SMTP server IP address" {
                  n298 = local write "SMTP server IP address"(w568) -> ()
                  n299 = global write "Preference_global.vi" "SMTP server IP address"(w568) -> ()
                }
                frame "Server Comms" {
                  n300 = Equal?(x="TRUE", y=w571) -> (x = y?=w570:bool)
                  n301 = case shown="False" w570 {
                    tunnel: [Server_Comms."Do Not Link To Server" ("Server Comms") Server_Comms."Server Link Healthy" ("Server Comms")] -> w569
                    frame False {
                    }
                    frame True {
                    }
                  }
                  n302 = local write "Server Comms"(w569) -> ()
                  n303 = global write "Preference_global.vi" "Server Comms"(w569) -> ()
                }
                frame "Temperature" {
                  n304 = global write "Preference_global.vi" "Temperature"(w575) -> ()
                  n305 = local write "Temperature"(w575) -> ()
                }
                frame "Abs Press (mbar)" {
                  n306 = global write "Preference_global.vi" "Abs Press (mbar)"(w576) -> ()
                  n307 = local write "Abs Press (mbar)"(w576) -> ()
                }
                frame "Qnet Site Root" {
                  n308 = String To Path(string=w578) -> (path=w577:path)
                  n309 = global write "Qnet_Globals.vi" "Local Site Root"(w577) -> ()
                  n310 = local write "Qnet Site Root"(w577) -> ()
                }
                frame "Current Overhead Factor" {
                  n311 = Fract/Exp String To Number(string=w580) -> (number=w579:dbl)  [unwired: 4 out]
                  n312 = call "Overhead_Factor.vi"("Current Overhead Factor In"=w579, "Mode"=Overhead."Initialise totals to 3hr") -> ()  [unwired: 2 in, 1 out]
                }
                frame "Auto Calib Error fr Previous" {
                  n313 = Fract/Exp String To Number(string=w583) -> (number=w582:dbl)  [unwired: 4 out]
                  n314 = global write "Preference_global.vi" "% Error From Previous Calib"(w582) -> ()
                  n315 = local write "% Error From Previous Calib"(w582) -> ()
                }
                frame "Auto Calib Error fr First" {
                  n316 = Fract/Exp String To Number(string=w585) -> (number=w584:dbl)  [unwired: 4 out]
                  n317 = global write "Preference_global.vi" "% Error From First Calib"(w584) -> ()
                  n318 = local write "% Error From First Calib"(w584) -> ()
                }
              }
            }
            frame "Char not in string" {
            }
          }
        }
        n319 = local read "Post Processing Machine"() -> (w539:bool)
        n320 = Select(t="Check file permission status", s=w539, f="is traverse setup blank?") -> (s? t:f=w537:string)
        n321 = Build Array (concatenate)(w541, w533) -> (w540:path[])
      }
      frame "is traverse setup blank?" {
        n322 = local read "Data Folder"() -> (w592:path)
        n323 = global read "Trav_pos_global.vi" "Default Traverse Setup"() -> (w586:string)
        n324 = Build Path(base path=w592, name or relative path="Preferences") -> (appended path=w591:path)
        n325 = Build Path(base path=w591, name or relative path=w595) -> (appended path=w590:path)
        n326 = List Folder(path=w590) -> (folder names=w588:string[])  [unwired: 1 in, 5 out]
        n327 = Search 1D Array(1D array=w588, element=w586) -> (index of element=w589:i32)  [unwired: 1 out]
        n328 = case shown="0, Default" w589 {
          tunnel: w588 -> [_ w601]
          tunnel: [w599 w600] -> w587
          tunnel: w586 -> [w599 _]
          frame 0, Default {
          }
          frame -1 {
            n329 = Index Array(array=w601, index=0) -> (element=w600:string)
          }
        }
        n330 = global write "Trav_pos_global.vi" "Default Traverse Setup"(w587) -> ()
      }
      frame "Please Enter new  Traverse Setup" {
        n331 = global read "Trav_pos_global.vi" "Default Traverse Setup"() -> (w605:string)
        n332 = String Length(string=w605) -> (length=w610:i32)
        n333 = In Range and Coerce(upper limit=w607, x=w610, lower limit=w608) -> (In Range?=w606:bool)  [unwired: 1 out]
        n334 = case shown="False" w606 {
          tunnel: w605 -> [w621 w629]
          tunnel: ["Please Enter new  Traverse Setup" "Update Traverse setup menu ring"] -> w609
          tunnel: [w614 w629] -> w604
          tunnel: w608 -> [w618 _]
          tunnel: w607 -> [w617 _]
          frame False {
            n335 = Format Into String(format string="Please Enter a Traverse Setup Name\nIt must be between %d and %d Characters" ("Message to user"), w618, w617) -> (resulting string=w616:string)  [unwired: 2 in, 1 out]
            n336 = call "Input_String_Dialog.vi"("Value"=w621, "Message to user"=w616) -> ("Ok Out"=w613:bool, "Output string"=w615:string)
            n337 = case shown="False" w613 {
              tunnel: w615 -> [_ w626]
              tunnel: [w622 w625] -> w614
              frame False {
                n338 = property on="Default Traverse Name" class="Ring (strict)"() -> ("Strings []"=w623:string[])  [unwired: 2 in, 2 out]
                n339 = Index Array(array=w623, index=0) -> (element=w622:string)
              }
              frame True {
                n340 = call "Fast_string_Replace.vi"("Replace match with:"="_", "Input String"=w626, "regular expression"=" ") -> ("Output String"=w625:string)  [unwired: 2 out]
              }
            }
          }
          frame True {
          }
        }
        n341 = global write "Trav_pos_global.vi" "Default Traverse Setup"(w604) -> ()
      }
      frame "Update Traverse setup menu ring" {
        n342 = global read "Trav_pos_global.vi" "Default Traverse Setup"() -> (w634:string)
        n343 = local read "Data Folder"() -> (w640:path)
        n344 = Build Path(base path=w640, name or relative path="Preferences") -> (appended path=w639:path)
        n345 = Build Path(base path=w639, name or relative path=w632) -> (appended path=w638:path)
        n346 = List Folder(path=w638) -> (folder names=w636:string[])  [unwired: 1 in, 5 out]
        n347 = Build Array (concatenate)(w636, "--New Traverse Setup--") -> (w635:string[])
        n348 = Search 1D Array(1D array=w635, element=w634) -> (index of element=w642:i32)  [unwired: 1 out]
        n349 = case shown="-1" w642 {
          tunnel: [w648 0] -> w644
          tunnel: w635 -> [w647 w651]
          tunnel: w634 -> [_ w650]
          tunnel: w642 -> [w648 _]
          tunnel: [w647 w649] -> w633
          frame 0, Default {
          }
          frame -1 {
            n350 = Build Array (concatenate)(w650, w651) -> (w649:string[])
          }
        }
        n351 = local write "Default Traverse Name"(w644) -> ()
        n352 = property on="Default Traverse Name" class="Ring (strict)"("Strings []"=w633) -> ()  [unwired: 2 in, 2 out]
      }
      frame "Create Traverse setup" {
        n353 = local read "Templates"() -> (w654:path)
        n354 = Build Path(base path=w654, name or relative path="All_Traverses") -> (appended path=w660:path)
        n355 = stacked-sequence {
          seq-local: [w665 _] -> [_ w693]
          seq-local: [w664 _] -> [_ _]
          tunnel: w660 -> [w667 _]
          tunnel: [w670 _] -> w657
          tunnel: [w669 _] -> w656
          tunnel: w654 -> [_ w692]
          tunnel: [_ w690] -> w653
          frame #0 {
            w673 = "Default_Space_file.xls" ("name or relative path")
            w668 = "Traverse_Setup.xls" ("name or relative path")
            n356 = global read "Trav_pos_global.vi" "Default Traverse Setup"() -> (w664:string)
            n357 = global read "Constants_global.vi" "Traverse folder"() -> (w677:path)
            n358 = Build Path(base path=w667, name or relative path=w673) -> (appended path=w671:path)
            n359 = Build Path(base path=w667, name or relative path=w668) -> (appended path=w666:path)
            n360 = Build Path(base path=w677, name or relative path=w664) -> (appended path=w665:path)
            n361 = Build Path(base path=w665, name or relative path="Trav_Space_Files") -> (appended path=w674:path)
            n362 = Build Path(base path=w674, name or relative path=w673) -> (appended path=w670:path)
            n363 = call "Does_file_exist_(simple).vi"("Pathname"=w670) -> ("exists?"=w672:bool)
            n364 = case shown="False" w672 {
              tunnel: w671 -> [w680 _]
              tunnel: w670 -> [w679 _]
              frame False {
                n365 = call "Create_directory_path.vi"("Path name"=w679) -> ("Path name Out"=w678:path)
                n366 = Copy(10:w678, 11:w680) -> ()  [unwired: 1 in, 5 out]
              }
              frame True {
              }
            }
            n367 = Build Path(base path=w665, name or relative path=w668) -> (appended path=w669:path)
            n368 = call "Does_file_exist_(simple).vi"("Pathname"=w669) -> ("exists?"=w676:bool)
            n369 = case shown="False" w676 {
              tunnel: w666 -> [w689 _]
              tunnel: w669 -> [w685 _]
              tunnel: w664 -> [w688 _]
              frame False {
                w681 = TRUE  # append to file? (new file:F)
                n370 = call "Create_directory_path.vi"("Path name"=w685) -> ("Path name Out"=w684:path)
                n371 = call "Read_File_Simple.vi"("Filename"=w689) -> ("string"=w687:string)  [unwired: 2 in, 7 out]
                n372 = call "Fast_string_Replace.vi"("Replace match with:"=w688, "Input String"=w687, "regular expression"="A_Tunnel") -> ("Output String"=w683:string)  [unwired: 2 out]
                n373 = call "Write_Characters_To_File.vi"("file path (dialog if empty)"=w684, "advisory dialog? (display:T)"=TRUE, "character string"=w683, "append to file? (new file:F)"=w681) -> ()  [unwired: 1 in, 4 out]
              }
              frame True {
              }
            }
          }
          frame #1 {
            w691 = "Traverse_Preferences.txt" ("name or relative path")
            n374 = Build Path(base path=w693, name or relative path=w691) -> (appended path=w690:path)
            n375 = Build Path(base path=w692, name or relative path=w691) -> (appended path=w694:path)
            n376 = call "Does_file_exist_(simple).vi"("Pathname"=w690) -> ("exists?"=w695:bool)
            n377 = case shown="False" w695 {
              tunnel: w694 -> [w698 _]
              tunnel: w690 -> [w697 _]
              frame False {
                n378 = call "Create_directory_path.vi"("Path name"=w697) -> ("Path name Out"=w696:path)
                n379 = Copy(10:w696, 11:w698) -> ()  [unwired: 1 in, 5 out]
              }
              frame True {
              }
            }
          }
        }
        n380 = Build Array (concatenate)(w659, w656, w653, w657) -> (w658:path[])
      }
      frame "Check file permission status" {
        n381 = local read "Post Processing Machine"() -> (w699:bool)
        n382 = for {
          tunnel: w704 -> [w718] mode=indexing
          shift-right: [w715] -> w701
          shift-left: "" -> [w716]
          n383 = call "Can_File_be_Editted.vi"("Filename"=w718) -> ("File Permissions OK?"=w719:bool, "Comment String"=w717:string)  [unwired: 2 out]
          n384 = case shown="False" w719 {
            tunnel: w718 -> [w724 _]
            tunnel: w717 -> [w723 _]
            tunnel: w716 -> [w722 w725]
            tunnel: [w721 w725] -> w715
            frame False {
              n385 = Format Into String(format string="\"%s\" %s\n", initial string=w722, w724, w723) -> (resulting string=w721:string)  [unwired: 1 in, 1 out]
            }
            frame True {
            }
          }
        }
        n386 = case shown="\"Load, Edit then Save\"" w705 {
          tunnel: [w727 w731] -> w706
          tunnel: w699 -> [w726 w730]
          frame "Save Preferences to file", Default {
            n387 = Select(t="Save Preference File", s=w726, f="Output Dev Number") -> (s? t:f=w727:string)
          }
          frame "Load, Edit then Save" {
            n388 = Select(t="Data Folder Changed?", s=w730, f="What next1") -> (s? t:f=w731:string)
          }
        }
        n389 = Empty String/Path?(string/path=w701) -> (empty?=w702:bool)
        n390 = case shown="True" w702 {
          tunnel: w701 -> [w714 _]
          frame False {
            n391 = Concatenate Strings("The following file permissions need to be sorted out before the software will run correctly.\n\n" ("string"), w714) -> (w712:string)
            n392 = Two Button Dialog(message=w712, 1:"Continue" ("F button name (\"Cancel\")"), 2:"Abort" ("F button name (\"Cancel\")")) -> (T button?=w709:bool)
            n393 = Stop(stop? (T)=w709) -> ()
          }
          frame True {
          }
        }
      }
      frame "What next1" {
        n394 = property on="Rig Setup" class="Ring (strict)"() -> ("Strings []"=w736:string[])  [unwired: 2 in, 2 out]
        n395 = Array Size(array=w736) -> (size(s)=w740:i32)
        n396 = Decrement(x=w740) -> (x-1=w739:i32)
        n397 = Equal?(x=w739, y="Rig Setup") -> (x = y?=w738:bool)
        n398 = case shown="False" w738 {
          tunnel: [w744 "Please Enter New Rig Name" ("t")] -> w737
          tunnel: w736 -> [w747 _]
          tunnel: "Rig Setup" -> [w746 _]
          frame False {
            n399 = global read "Preference_global.vi" "Rig Setup"() -> (w748:string)
            n400 = Index Array(array=w747, index=w746) -> (element=w743:string)
            n401 = Not Equal?(x=w743, y=w748) -> (x != y?=w745:bool)
            n402 = case shown="False" w745 {
              tunnel: ["What next2" ("f") "Update Rig setup menu ring" ("t")] -> w744
              tunnel: w743 -> [_ w750]
              frame False {
              }
              frame True {
                n403 = global write "Preference_global.vi" "Rig Setup"(w750) -> ()
              }
            }
          }
          frame True {
            n404 = global write "Preference_global.vi" "Rig Setup"("") -> ()
          }
        }
      }
      frame "What next2" {
        n405 = property on="Default Traverse Name" class="Ring (strict)"() -> ("Strings []"=w756:string[])  [unwired: 2 in, 2 out]
        n406 = Array Size(array=w756) -> (size(s)=w760:i32)
        n407 = Decrement(x=w760) -> (x-1=w759:i32)
        n408 = Equal?(x=w759, y="Default Traverse Name") -> (x = y?=w758:bool)
        n409 = case shown="False" w758 {
          tunnel: [w764 "Please Enter new  Traverse Setup" ("t")] -> w757
          tunnel: w756 -> [w768 _]
          tunnel: "Default Traverse Name" -> [w767 _]
          frame False {
            n410 = global read "Trav_pos_global.vi" "Default Traverse Setup"() -> (w766:string)
            n411 = Index Array(array=w768, index=w767) -> (element=w763:string)
            n412 = Not Equal?(x=w763, y=w766) -> (x != y?=w765:bool)
            n413 = case shown="False" w765 {
              tunnel: ["Data Folder Changed?" ("f") "Update Traverse setup menu ring" ("t")] -> w764
              tunnel: w763 -> [_ w770]
              frame False {
              }
              frame True {
                n414 = global write "Trav_pos_global.vi" "Default Traverse Setup"(w770) -> ()
              }
            }
          }
          frame True {
            n415 = global write "Trav_pos_global.vi" "Default Traverse Setup"("") -> ()
          }
        }
      }
      frame "Data Folder Changed?" {
        w775 = "Please Select your data folder"
        n416 = global read "Constants_global.vi" "Data Folder"() -> (w782:path)
        n417 = local read "Data Folder"() -> (w783:path)
        n418 = property on="OK" class="Bool (strict)"("Visible"=TRUE) -> ()  [unwired: 2 in, 2 out]
        n419 = while {
          shift-right: [w792] -> _
          shift-left: _ -> [w791]
          tunnel: [w790] -> w777
          stop <- TRUE stop-if-true
          n420 = local read "Post Processing Machine"() -> (w792:bool)
          n421 = Not Equal?(x=w792, y=w791) -> (x != y?=w790:bool)
        }
        n422 = Not Equal?(x=w782, y=w783) -> (x != y?=w781:bool)
        n423 = Select(t=w775, s=w781, f="Has OK has been pressed?") -> (s? t:f=w774:string)
        n424 = case shown="True" w777 {
          tunnel: [w786 w788] -> w776
          tunnel: w775 -> [_ w788]
          tunnel: w774 -> [w786 _]
          frame False {
          }
          frame True {
            n425 = global write "Preference_global.vi" "Rig Setup"("") -> ()
          }
        }
      }
      frame "Has OK has been pressed?" {
        n426 = flat-sequence {
          tunnel: ["OK"] -> w794
          frame #0 {
            n427 = Wait (ms)(milliseconds to wait=u32 100) -> ()  [unwired: 1 out]
          }
          frame #1 {
          }
        }
        n428 = local read "Post Processing Machine"() -> (w795:bool)
        n429 = case shown="True" w794 {
          tunnel: w795 -> [w800 w806]
          tunnel: [w799 w803] -> w793
          frame False {
            n430 = Select(t="Data Folder Changed?", s=w800, f="What next1") -> (s? t:f=w799:string)
          }
          frame True {
            n431 = Select(t="Save Preference File", s=w806, f="Output Dev Number") -> (s? t:f=w803:string)
          }
        }
      }
      frame "Output Dev Number" {
        n432 = stacked-sequence {
          seq-local: [w814 _ _] -> [_ w850 _]
          tunnel: w811 -> [_ _ _]
          frame #0 {
            w817 = T11 0 items=["Canonical Names Only"=0, "Aliases Only"=1, "Include Matching Aliases"=2, "Include All Aliases"=4] ("Search Mode")
            n433 = VISA Find Resource(10:w817) -> (3:w816:string[])  [unwired: 1 in, 3 out]
            n434 = for {
              shift-right: [w832] -> w814
              shift-left: string[] [] -> [w833]
              tunnel: w816 -> [w822] mode=indexing
              n435 = Reverse String(1:w822) -> (0:w830:string)
              n436 = Match Pattern(string=w830, regular expression="::") -> (before substring=w829:string)  [unwired: 4 out]
              n437 = Match Pattern(string=w822, regular expression="NI-VISA") -> (offset past match=w821:i32)  [unwired: 4 out]
              n438 = Reverse String(1:w829) -> (0:w827:string)
              n439 = Less Than 0?(x=w821) -> (x < 0?=w819:bool)
              n440 = Equal?(x=w827, y="INSTR") -> (x = y?=w825:bool)
              n441 = Equal?(x=w827, y="RAW") -> (x = y?=w824:bool)
              n442 = Or(x=w825, y=w824) -> (x .or. y?=w820:bool)
              n443 = And(x=w820, y=w819) -> (x .and. y?=w818:bool)
              n444 = case shown="True" w818 {
                tunnel: w833 -> [w834 w837]
                tunnel: [w834 w836] -> w832
                tunnel: w822 -> [_ w835]
                frame False {
                }
                frame True {
                  n445 = Build Array (concatenate)(w837, w835) -> (w836:string[])
                }
              }
            }
          }
          frame #1 {
            w842 = "Dev" ("format string")
            n446 = local read "Analogue Device Serial No."() -> (w846:string)
            n447 = String Length(string=w842) -> (length=w844:i32)
            n448 = local read "PWA Device Serial No."() -> (w840:string)
            n449 = String Subset(string=w846, length (rest)=w844) -> (substring=w848:string)  [unwired: 1 out]
            n450 = String Subset(string=w840, length (rest)=w844) -> (substring=w843:string)  [unwired: 1 out]
            n451 = Equal?(x=w848, y=w842) -> (x = y?=w845:bool)
            n452 = Equal?(x=w842, y=w843) -> (x = y?=w841:bool)
            n453 = for {
              tunnel: w846 -> [w869]
              tunnel: w850 -> [w867] mode=indexing
              tunnel: [w868] -> w862 mode=indexing
              tunnel: w840 -> [w866]
              tunnel: [w865] -> w859 mode=indexing
              n454 = Match Pattern(string=w867, regular expression=w869) -> (offset past match=w868:i32)  [unwired: 1 in, 3 out]
              n455 = Match Pattern(string=w867, regular expression=w866) -> (offset past match=w865:i32)  [unwired: 1 in, 3 out]
            }
            n456 = Array Max & Min(array=w862) -> (max index (indices)=w863:i32)  [unwired: 3 out]
            n457 = Array Max & Min(array=w859) -> (max index (indices)=w861:i32)  [unwired: 3 out]
            n458 = Increment(x=w861) -> (x+1=w852:i32)
            n459 = Increment(x=w863) -> (x+1=w856:i32)
            n460 = Equal To 0?(x=w856) -> (x = 0?=w858:bool)
            n461 = Equal To 0?(x=w852) -> (x = 0?=w853:bool)
            n462 = Select(t=1, s=w858, f=w856) -> (s? t:f=w857:i32)
            n463 = Select(t=1, s=w853, f=w852) -> (s? t:f=w851:i32)
            n464 = Format Into String(format string="Dev%d", w857) -> (resulting string=w847:string)  [unwired: 2 in, 1 out]
            n465 = Format Into String(format string="Dev%d", w851) -> (resulting string=w839:string)  [unwired: 2 in, 1 out]
            n466 = Select(t=w846, s=w845, f=w847) -> (s? t:f=w849:string)
            n467 = Select(t=w840, s=w841, f=w839) -> (s? t:f=w838:string)
            n468 = global write "PWAtasksGLOBAL.vi" "Analogue Dev Name"(w849) -> ()
            n469 = global write "PWAtasksGLOBAL.vi" "PWA Dev Name"(w838) -> ()
          }
          frame #2 {
            n470 = for {
              tunnel: string[] ["Raw_Calibrations", "Raw_Measurements", "Results", "Calibrations", "Commands"] -> [w874] mode=indexing
              n471 = call "Data_folder_Path.vi"("Data Type"=w874) -> ("Data Folder"=w873:path)  [unwired: 4 in]
              n472 = Build Path(base path=w873, name or relative path="Test" ("Substring")) -> (appended path=w876:path)
              n473 = call "Create_directory_path.vi"("Path name"=w876) -> ()  [unwired: 1 out]
            }
            n474 = call "Data_folder_Path.vi"("Data Type"="Results_Post_Processed" ("element")) -> ("Data Folder"=w870:path)  [unwired: 4 in]
            n475 = call "Create_directory_path.vi"("Path name"=w870) -> ()  [unwired: 1 out]
          }
        }
      }
      frame "Save Preference File" {
        n476 = call "Date_and_Time_to_string.vi"() -> ("Date and time (spreadsheet)"=w888:string)
        n477 = call "Setup_Filepath.vi"("Setup File Type"=Setup_Filetype."General", "Filename in"=w878) -> ("Filename Out"=w877:path)  [unwired: 1 out]
        n478 = for {
          tunnel: w887 -> [w898] mode=indexing
          shift-right: [w894] -> w886
          shift-left: w888 -> [w896]
          n479 = case shown="\"Analogue Device Serial No.\"" w898 {
            tunnel: w898 -> [w901 _ _ _ _ _ _ _ _ _ _ _ _ _ _ _ _]
            tunnel: ["No Match" "Server address" w904 w906 w908 w912 "SMTP server IP address" "PWA Device Serial No." "Analogue Device Serial No." w916 w918 "Temperature" "Abs Press (mbar)" w923 w928 w931 w934] -> w897
            frame "No Match", Default {
              n480 = call "Was_string_matched.vi"("Match Error"=TRUE, "Variable name"=w901) -> ()  [unwired: 1 in]
            }
            frame "Server address" {
              n481 = global write "Preference_global.vi" "Server address"("Server address") -> ()
            }
            frame "Server port number" {
              n482 = global write "Preference_global.vi" "Server port number"("Server port number") -> ()
              n483 = Number To Decimal String(number="Server port number") -> (decimal integer string=w904:string)  [unwired: 1 out]
            }
            frame "Default Source Establishment Time (s)" {
              n484 = global write "Preference_global.vi" "Default Source Establishment Time (s)"("Default Source Establishment Time (s)") -> ()
              n485 = Number To Decimal String(number="Default Source Establishment Time (s)") -> (decimal integer string=w906:string)  [unwired: 1 out]
            }
            frame "Tunnel Speed Control" {
              n486 = global write "Preference_global.vi" "Tunnel Speed Control"("Tunnel Speed Control") -> ()
              n487 = Select(t="TRUE", s="Tunnel Speed Control", f="FALSE") -> (s? t:f=w908:string)
            }
            frame "LabVIEW Administrators" {
              n488 = global write "Preference_global.vi" "LabVIEW Administrators"("LabVIEW Administrators") -> ()
              n489 = call "Put_Array_into_String.vi"("String array"="LabVIEW Administrators") -> ("String Value"=w912:string)
            }
            frame "SMTP server IP address" {
              n490 = global write "Preference_global.vi" "SMTP server IP address"("SMTP server IP address") -> ()
            }
            frame "PWA Device Serial No." {
            }
            frame "Analogue Device Serial No." {
            }
            frame "Default Traverse Name" {
              n491 = global read "Trav_pos_global.vi" "Default Traverse Setup"() -> (w916:string)
            }
            frame "Server Comms" {
              n492 = case shown="\"Server Link Healthy\"" "Server Comms" {
                tunnel: ["TRUE" "FALSE"] -> w918
                frame "Server Link Healthy" {
                }
                frame "Do Not Link To Server" {
                }
              }
              n493 = global write "Preference_global.vi" "Server Comms"("Server Comms") -> ()
            }
            frame "Temperature" {
              n494 = global write "Preference_global.vi" "Temperature"("Temperature") -> ()
            }
            frame "Abs Press (mbar)" {
              n495 = global write "Preference_global.vi" "Abs Press (mbar)"("Abs Press (mbar)") -> ()
            }
            frame "Current Overhead Factor" {
              n496 = call "Overhead_Factor.vi"("Mode"=Overhead."Read Current Overhead") -> ("Current Overhead Factor"=w925:dbl)  [unwired: 3 in]
              n497 = Number To Fractional String(number=w925, precision (6)=i16 4) -> (F-format string=w923:string)  [unwired: 2 out]
            }
            frame "Auto Calib Error fr Previous" {
              n498 = global write "Preference_global.vi" "% Error From Previous Calib"("% Error From Previous Calib") -> ()
              n499 = Number To Fractional String(number="% Error From Previous Calib", precision (6)=i16 2) -> (F-format string=w928:string)  [unwired: 2 out]
            }
            frame "Auto Calib Error fr First" {
              n500 = global write "Preference_global.vi" "% Error From First Calib"("% Error From First Calib") -> ()
              n501 = Number To Fractional String(number="% Error From First Calib", precision (6)=i16 2) -> (F-format string=w931:string)  [unwired: 2 out]
            }
            frame "Qnet Site Root" {
              n502 = global write "Qnet_Globals.vi" "Local Site Root"("Qnet Site Root") -> ()
              n503 = Path To String(path="Qnet Site Root") -> (string=w934:string)
            }
          }
          n504 = call "Characters_to_string.vi"("Characters to write"=w897, "Label for characters"=w898) -> ("Output string"=w895:string)
          n505 = Concatenate Strings(w896, w895) -> (w894:string)
        }
        n506 = case shown="\"Load, Edit then Save\"" w882 {
          tunnel: [TRUE TRUE TRUE] -> w881
          frame "Load, Edit then Save" {
            n507 = Current VI's Path() -> (path=w890:path)
            n508 = call "Open_Close_Front_Panel.ph.vi"("Front Panel Window:Open"=FALSE, "VI path"=w890) -> ()  [unwired: 2 out]
          }
          frame "Load Preferences from file" {
          }
          frame "Save Preferences to file" {
          }
        }
        n509 = call "Write_Characters_To_File.vi"("file path (dialog if empty)"=w877, "advisory dialog? (display:T)"=FALSE, "character string"=w886, "append to file? (new file:F)"=FALSE) -> ()  [unwired: 1 in, 4 out]
      }
      frame "Save SW Preferences" {
        w950 = FALSE  # append to file? (new file:F)
        w951 = FALSE  # advisory dialog? (display:T)
        n510 = local read "Post Processing Machine"() -> (w940:bool)
        n511 = Path To String(path="Data Folder") -> (string=w942:string)
        n512 = global read "Preference_global.vi" "Server Comms"() -> (w946:T2)
        n513 = call "Characters_to_string.vi"("Characters to write"=w942, "Label for characters"=w944) -> ("Output string"=w952:string)
        n514 = Select(t="True", s=w940, f="False") -> (s? t:f=w937:string)
        n515 = call "Characters_to_string.vi"("Characters to write"=w937, "Label for characters"=w935) -> ("Output string"=w936:string)
        n516 = call "Date_and_Time_to_string.vi"() -> ("Date and time (spreadsheet)"=w947:string)
        n517 = case shown="\"Server Link Healthy\"" w946 {
          tunnel: ["Update Served VI file" "Update Local Adam Table"] -> w945
          frame "Server Link Healthy" {
          }
          frame "Do Not Link To Server" {
          }
        }
        n518 = Concatenate Strings(w947, w952, w936) -> (w948:string)
        n519 = local read "EnFlo SW Preferences"() -> (w949:path)
        n520 = call "Write_Characters_To_File.vi"("file path (dialog if empty)"=w949, "advisory dialog? (display:T)"=w951, "character string"=w948, "append to file? (new file:F)"=w950) -> ()  [unwired: 1 in, 4 out]
      }
      frame "Update Local Adam Table" {
        n521 = stacked-sequence {
          seq-local: [w966 _] -> [_ w980]
          tunnel: ["Update Served VI file" _] -> w958
          frame #0 {
            w966 = T12 {"Ch Name"="", "Type"=enum."4011", "Function"=enum."Analogue Input", "Ch State"=enum."On", "Calibration type"=enum."Raw", "A"=0.0, "B"=0.0, "C"=0.0, "D"=0.0, "Comments"="", "Address"={"Main"=0, "Ch."=0, "Sub"=0, "Port Name"=""}, "String"="", "Duty"=0} ("Ch Discription")
            n522 = global read "Preference_global.vi" "Abs Press (mbar)"() -> (w963:string)
            n523 = global read "Preference_global.vi" "Temperature"() -> (w964:string)
            n524 = Bundle By Name(cluster=w966, "Type"=Module_type_ADAM."Hold Value", "Calibration type"=Calib_type_ADAM."Raw", "A"=1.0) -> (w967:T12)
            n525 = Build Array(w964, w963) -> (w962:string[])
            n526 = for {
              tunnel: [w973] -> w965 mode=indexing
              tunnel: w967 -> [w972]
              tunnel: w962 -> [w971] mode=indexing
              n527 = Bundle By Name(cluster=w972, "Ch Name"=w971) -> (w973:T12)
            }
            n528 = call "Update_Ch_Discription_client.vi"("Channels to update In"=w965) -> ()  [unwired: 1 out]
          }
          frame #1 {
            n529 = global read "Preference_global.vi" "Rig Setup"() -> (w975:string)
            n530 = call "Get_Current_Scan_client.vi"() -> ("Ch Description Array"=w981:T12[])  [unwired: 1 in, 3 out]
            n531 = Match Pattern(string=w975, regular expression="-") -> (before substring=w974:string)  [unwired: 4 out]
            n532 = Format Into String(format string="%s Metadata:" ("Format String"), w974) -> (resulting string=w983:string)  [unwired: 2 in, 1 out]
            n533 = Initialize Array(w980, 0 ("dimension size")) -> (w978:T12[])
            n534 = for {
              shift-right: [w994] -> w977
              shift-left: w978 -> [w995]
              tunnel: w981 -> [w986] mode=indexing
              tunnel: w983 -> [w993]
              tunnel: "Metadata:" ("Format String") -> [w992]
              n535 = Unbundle By Name(w986) -> ("Ch Name"=w985:string)
              n536 = Match Pattern(string=w985, regular expression=w993) -> (offset past match=w990:i32)  [unwired: 4 out]
              n537 = Match Pattern(string=w985, regular expression=w992) -> (offset past match=w991:i32)  [unwired: 4 out]
              n538 = Greater Or Equal To 0?(x=w991) -> (x >= 0?=w988:bool)
              n539 = Less Than 0?(x=w990) -> (x < 0?=w989:bool)
              n540 = And(x=w989, y=w988) -> (x .and. y?=w987:bool)
              n541 = case shown="True" w987 {
                tunnel: w995 -> [w996 w1001]
                tunnel: [w996 w1000] -> w994
                tunnel: w986 -> [_ w999]
                frame False {
                }
                frame True {
                  n542 = Bundle By Name(cluster=w999, "Ch State"=Channel_State."Off") -> (w997:T12)
                  n543 = Build Array (concatenate)(w1001, w997) -> (w1000:T12[])
                }
              }
            }
            n544 = call "Update_Ch_Discription_client.vi"("Channels to update In"=w977) -> ()  [unwired: 1 out]
          }
        }
      }
      frame "Update Served VI file" {
        # "Template"
        # "Orig"
        n545 = call "Setup_Filepath.vi"("Setup File Type"=Setup_Filetype."General", "Filename in"=w1003) -> ("Filename Out"=w1002:path)  [unwired: 1 out]
        n546 = Build Array("Served:VI:Name", "Served:VI:Path", "Server:IP Number:& Port No") -> (w1008:string[])
        n547 = stacked-sequence {
          seq-local: [w1013 _ _ _] -> [_ _ w1023 _]
          seq-local: [_ w1020 _ _] -> [_ _ w1024 _]
          seq-local: [_ _ w1025 _] -> [_ _ _ w1050]
          tunnel: w1008 -> [w1015 w1021 _ w1051]
          tunnel: w1002 -> [w1014 _ _ w1052]
          tunnel: w1003 -> [_ w1017 _ _]
          frame #0 {
            n548 = call "Read_Ch_data_file.vi"("Present Channels"=w1015, "Output"=enum16{"All Ch data", "The last few rows"}."All Ch data", "Filename"=w1014) -> ("Channel Values"=w1013:string[][])  [unwired: 2 in, 4 out]
          }
          frame #1 {
            n549 = local read "Templates"() -> (w1019:path)
            n550 = Build Path(base path=w1019, name or relative path=w1017) -> (appended path=w1018:path)
            n551 = call "Read_Ch_data_file.vi"("Present Channels"=w1021, "Output"=enum16{"All Ch data", "The last few rows"}."All Ch data", "Filename"=w1018) -> ("Channel Values"=w1020:string[][])  [unwired: 2 in, 4 out]
          }
          frame #2 {
            n552 = Index Array(array=w1023, index (col)=0 ("Index")) -> (element=w1028:string[])  [unwired: 1 in]
            n553 = To Upper Case(1:w1024) -> (0:w1026:string[][])
            n554 = To Upper Case(1:w1028) -> (0:w1027:string[])
            n555 = for {
              tunnel: w1027 -> [w1031]
              tunnel: w1024 -> [w1036] mode=indexing
              tunnel: w1026 -> [w1030] mode=indexing
              tunnel: [w1033] -> w1025 mode=indexing
              tunnel: w1023 -> [w1032]
              n556 = Index Array(array=w1030, index=0 ("Index")) -> (element=w1034:string)
              n557 = Search 1D Array(1D array=w1031, element=w1034) -> (index of element=w1035:i32)  [unwired: 1 out]
              n558 = case shown="0, Default" w1035 {
                tunnel: w1036 -> [w1045 w1046]
                tunnel: w1035 -> [w1042 _]
                tunnel: [w1038 w1046] -> w1033
                tunnel: w1032 -> [w1043 _]
                frame 0, Default {
                  n559 = Index Array(array=w1043, index (row)=w1042, index (col)=2 ("Index")) -> (element=w1040:string)
                  n560 = Array Subset(array=w1045, length=2) -> (w1039:string[])  [unwired: 1 in]
                  n561 = Build Array (concatenate)(w1039, w1040) -> (w1038:string[])
                }
                frame -1 {
                }
              }
            }
          }
          frame #3 {
            w1047 = FALSE  # Append last row only
            w1048 = FALSE  # Lock File
            w1049 = FALSE  # exists?
            n562 = call "Write_Ch_data_file.vi"("Append last row only"=w1047, "Lock File"=w1048, "exists?"=w1049, "Channel Values"=w1050, "Channel names"=w1051, "Filename"=w1052) -> ()  [unwired: 2 in, 4 out]
          }
        }
      }
      frame "Initialise Globals" {
        w1057 = TRUE  # OK
        w1061 = FALSE  # append to file? (new file:F)
        w1060 = FALSE  # advisory dialog? (display:T)
        n563 = global read "Constants_global.vi" "ADAM setups folder"() -> (w1067:path)
        n564 = global read "Constants_global.vi" "All_Users"() -> (w1056:path)
        n565 = property on="ADAM Setup File" class="Ring (strict)"() -> ("Strings []"=w1062:string[])  [unwired: 2 in, 2 out]
        n566 = Build Path(base path=w1056, name or relative path="Current_Username") -> (appended path=w1054:path)
        n567 = Build Path(base path=w1067, name or relative path="Setup_Files") -> (appended path=w1065:path)
        n568 = global read "Preference_global.vi" "User_Name"() -> (w1053:string)
        n569 = Build Path(base path=w1065, name or relative path="Selected_Filename.txt" ("Substring")) -> (appended path=w1058:path)
        n570 = call "Get_users_email_addresses.vi"("OK"=w1057) -> ()  [unwired: 5 out]
        n571 = Index Array(array=w1062, index="ADAM Setup File") -> (element=w1059:string)
        n572 = call "Write_File_Simple.vi"("character string"=w1053, "file path"=w1054) -> ()  [unwired: 1 in, 2 out]
        n573 = global write "Dynamic_call_global.ph.vi" "Acquisition Interlock"(FALSE ("Acquisition Interlock")) -> ()
        n574 = call "Write_Characters_To_File.vi"("file path (dialog if empty)"=w1058, "advisory dialog? (display:T)"=w1060, "character string"=w1059, "append to file? (new file:F)"=w1061) -> ()  [unwired: 1 in, 4 out]
      }
    }
  }
  n575 = call "Get_IP_Number.vi"() -> ("IP Number"=→"This Machine's IP Number":string)
